vi "Wind_Turbine_1.vi"() -> (5 "Plug in titles":string[](array[string]), 7 "Plug in values":string[](array[string]))   [LabVIEW 2011]
uses:
  Controls/Analysis_info_cluster.ctl
  Controls/Inst_type.ctl
  Controls/Instrument_Array.ctl
  Controls/XY_Plot_Cluster.ctl
  Globals/Meas_global.vi
  Globals/LDA_meas_global_1.vi
  Plug in sub vis/Wind_Turbine_Global.vi
  Globals/Plug_in_data_global.vi
  <vilib>/Analysis/NI_AALBase.lvlib
  <vilib>/Analysis/NI_AALPro.lvlib
panel:
  in  "precision 2":string="3"
  in  "Separation Character 2":string="\t"
  out "L Status Phase lock index 2":i32
  out "Laser Phase lock index 2":i32
  out "XY Graph":cluster{dbl[], dbl[]}[](graph)
  out "WT Revolution Start times":dbl[](array[numeric])
  out "Angle 3":dbl format="%#_3g"
  out "Angle 2":dbl format="%#_3g"
  out "Angle 1":dbl format="%#_3g"
  out "L Status Phase lock index":i32
  out "Laser Status Index":i32
  out "Waveform Graph 3":dbl[](graph)
  out "Laser Phase lock index":i32
  out "Laser Disp Index":i32
  out "Av Variance 3":dbl
  out "Av Variance 2":dbl
  out "Av Variance 1":dbl
  out "slope 3":dbl format="%#_3g"
  out "slope 2":dbl format="%#_3g"
  out "Variance Blade 3":dbl[](graph)
  out "Variance Blade 2":dbl[](graph)
  out "Mean Blade 3":dbl[](graph)
  out "Mean Blade 2":dbl[](graph)
  out "Variance Blade 1":dbl[](graph)
  out "Av Disp 3":dbl
  out "Av Disp 2":dbl
  out "Av Disp 1":dbl
  out "slope 1":dbl format="%#_3g"
  in  "End Cut Deg":dbl
  in  "Start Cut Deg":dbl
  out "Waveform Graph 2":i16[](graph)
  out "Mean Blade 1":dbl[](graph)
  out "Array":i32[](array[numeric])
  in  "Angular Step":dbl=10.0
  in  "Turbine to Phase Lock to":u16(ring) items=["RV (WT1)"]
  in  "Change Dem Voltages?":bool=TRUE
  out "All WTs":dbl[][](array[numeric]) format="%#.2g"
  out "WT trace index":dbl[][](array[numeric])
  in  "precision":string
  in  "Add Phase data to results file":bool
  in  "Separation Character":string="\t"
  in  "Output Directory":path
  in  "Save Phase averaged Profiles":bool
  out "LDA Chs":i32[](array[numeric])
  out "WT Stalled?":bool
  out "Pulse No":i32
  out "Last index":i32
  out "subarray":bool[](array[boolean])
  out "Index":i32[](array[numeric])
  out "Pulses per Rev":i32
  out "Av samples per pulse":i32
  out "Threshold":dbl
  in  "Channel to Phase lock":i32[](listbox)
  out "Last Block No of Revs":i32
  out "Number of Revs":i32
  # "Mean RPM      SD RPM           Max-Min"
  # "Scroll down for Blade angle stats"
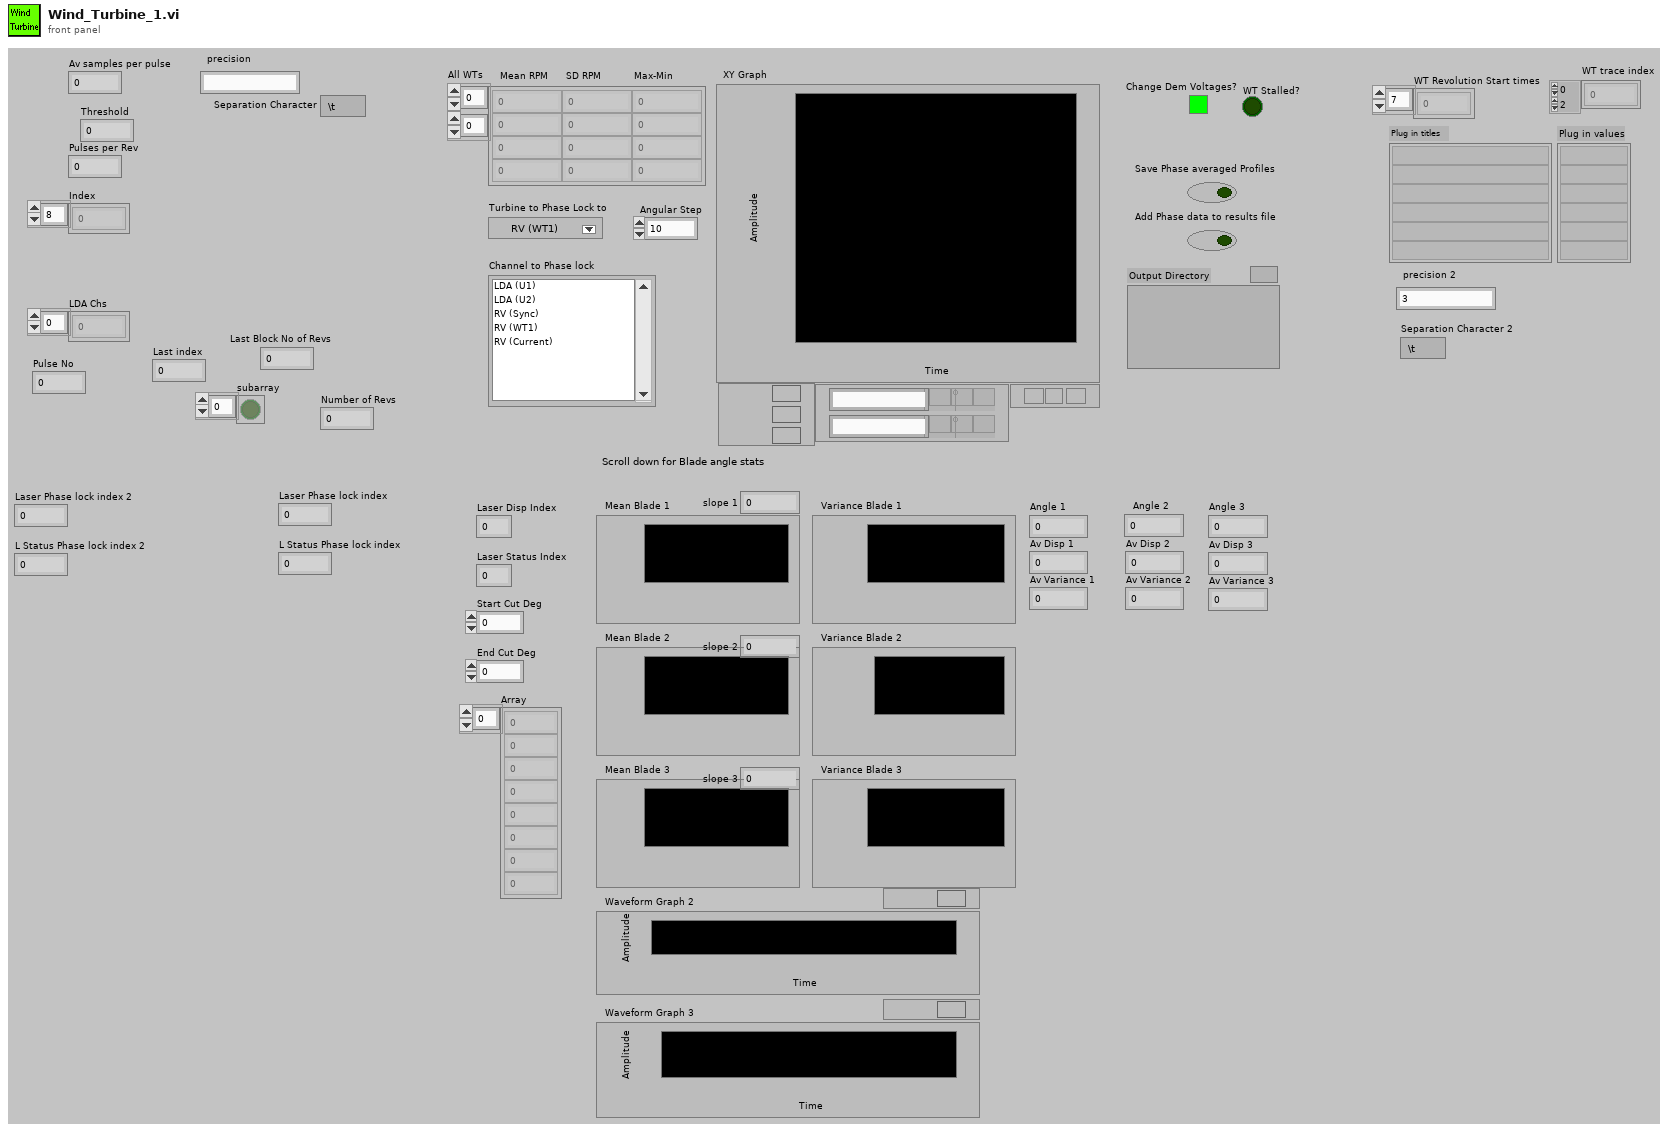
[diagram p1: front panel]
types:
  T1 = typedef "Analysis_info_cluster.ctl" = cluster{"Colour":u32, "Inst type":T2, "Inst name":string, "Symbol":string, "Code name":string, "Extra Info":string, "Inst Array":T3, "Extra Titles":string[], "Extra Values":string[], "Eng Values":dbl[], "Time (ms)":dbl[], "Voltage":dbl[], "U":dbl, "u^2":dbl, "u^3":dbl, "u^4":dbl, "Skew_u":dbl, "Kurt_u":dbl, "Sd Error in Mean":dbl, "% u'/U":dbl, "X":dbl, "Y":dbl, "Z":dbl, "Spectra":T4, "Autocorrelation":T4, "Timescale integral to 25%":dbl, "Sd Error in Variance":dbl, "Calib File":path, "Calib Constants":dbl[], "Histogram":T4, "Output Position":bool, "Full Stats":bool, "Weighting":dbl[], "Av Sampling Rate":dbl, "Av No of Samples":dbl, "Total Meas Time (s)":dbl}
  T2 = typedef "Inst_type.ctl" = enum16{"Propeller anemometer", "Raw voltage", "Pressure Transducer", "Pitot-static tube", "Preston tube", "Hot wire", "Cross wire 1", "Cross wire 2", "Generic Linear", "Generic Polynomial", "Generic BackPoly", "Fast FID", "Thermocouple", "Cold wire", "Pulsed Wire", "LDA Vel", "LDA Tran time", "LDA Arr time"}
  T3 = typedef "Instrument_Array.ctl" = enum16{"PWA", "LDA", "Analogue"}
  T4 = typedef "XY_Plot_Cluster.ctl" = cluster{"First Name":string, "Second Name":string, "X axis name":string, "Y axis name":string, "X array":dbl[], "Y array":dbl[]}
  T5 = typedef "Post_Process.ctl" = enum16{"Take New Data", "Post Process Raw Data File"}
  T6 = cluster{"[0]":bool, "[1]":bool, "[2]":bool, "[3]":bool}
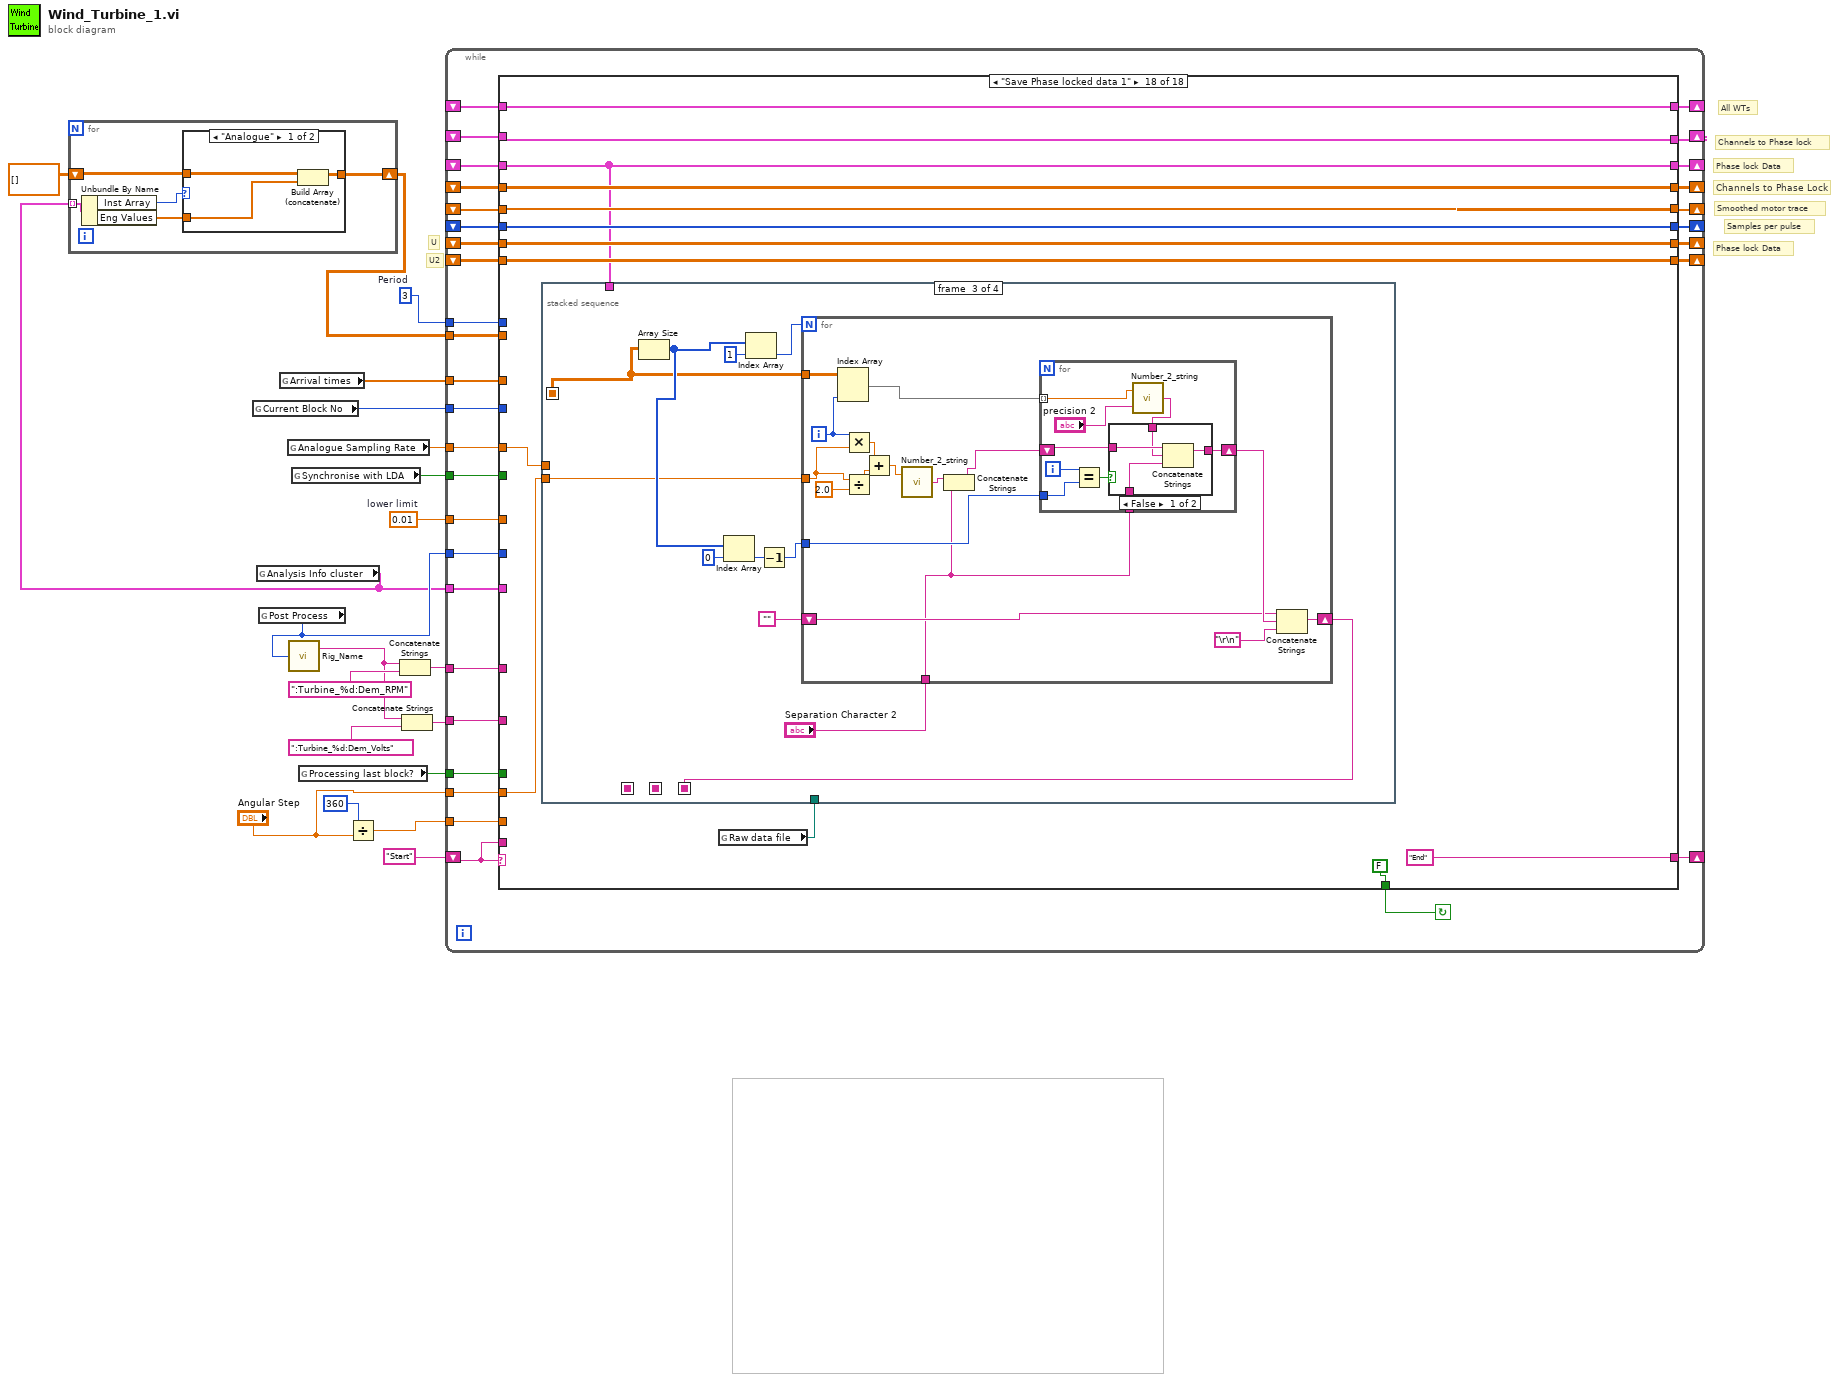
[diagram p0: block diagram]
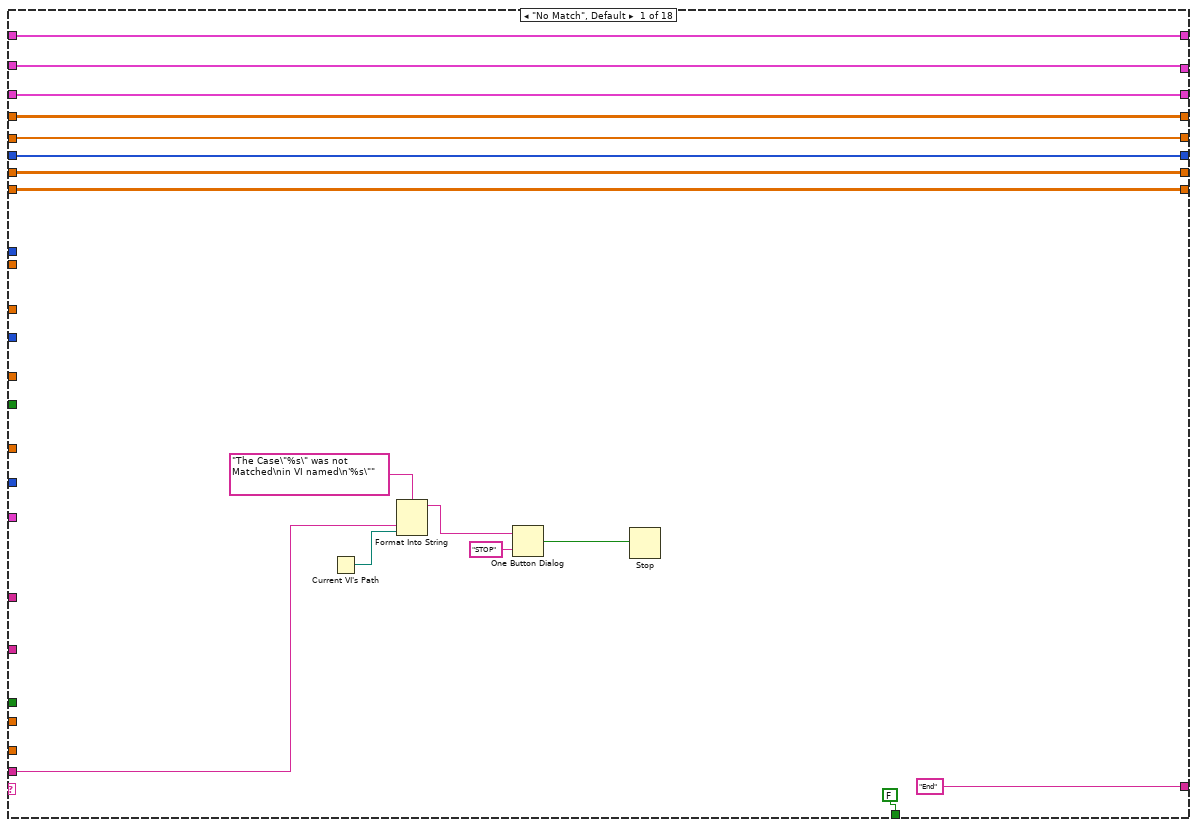
[diagram p3: hidden frame]
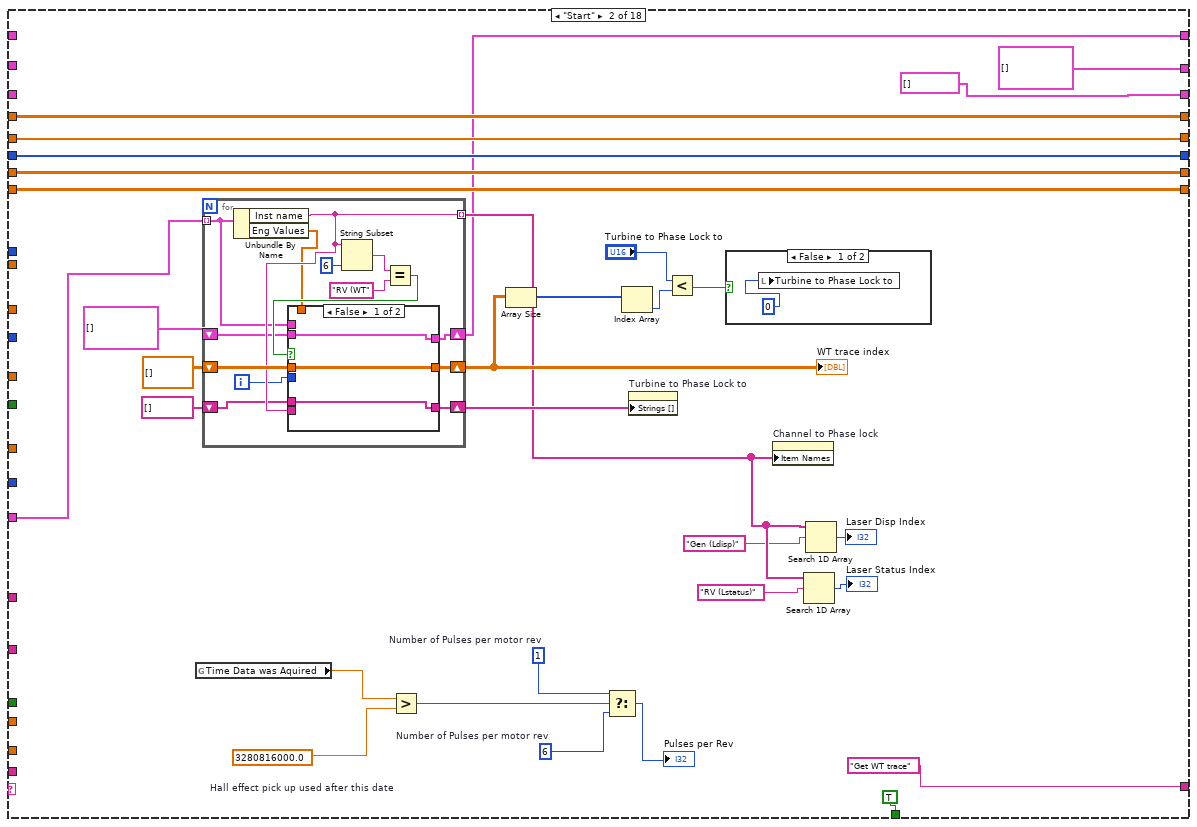
[diagram p4: hidden frame]
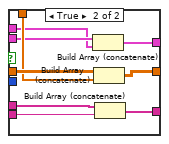
[diagram p6: hidden frame]
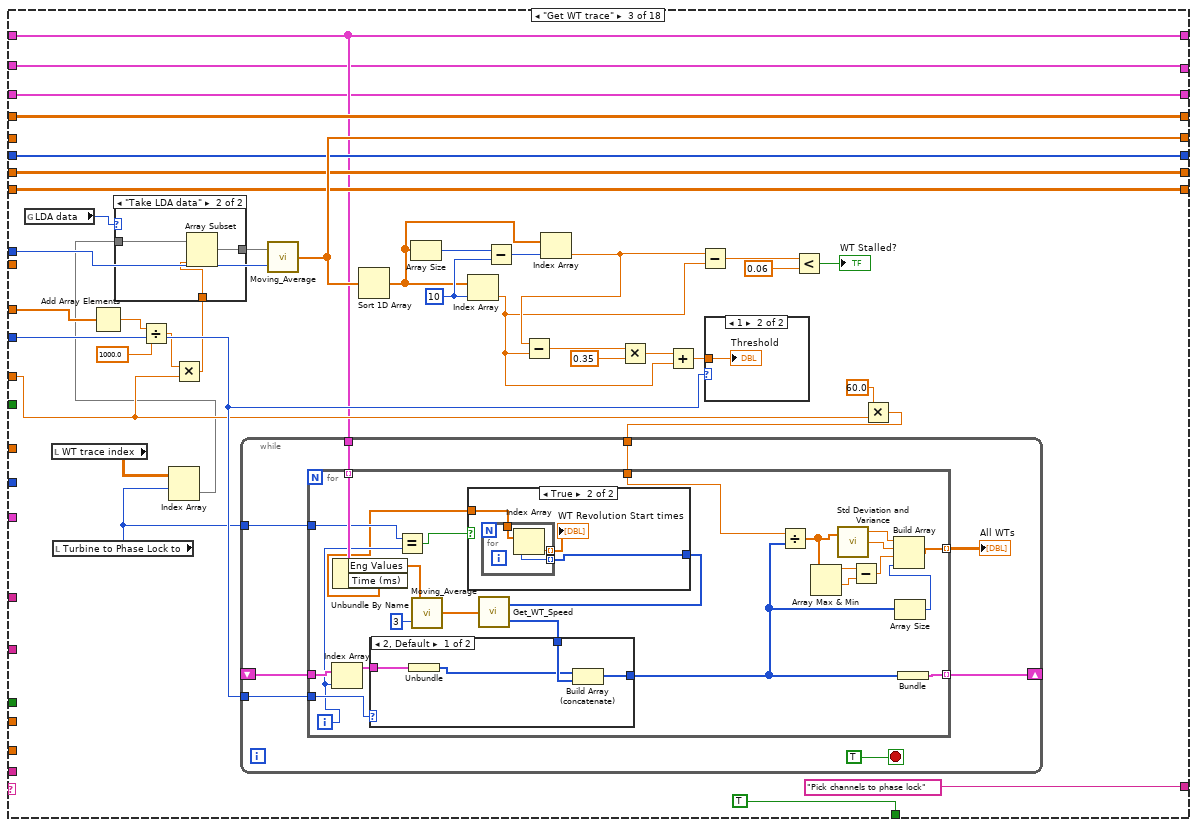
[diagram p7: hidden frame]
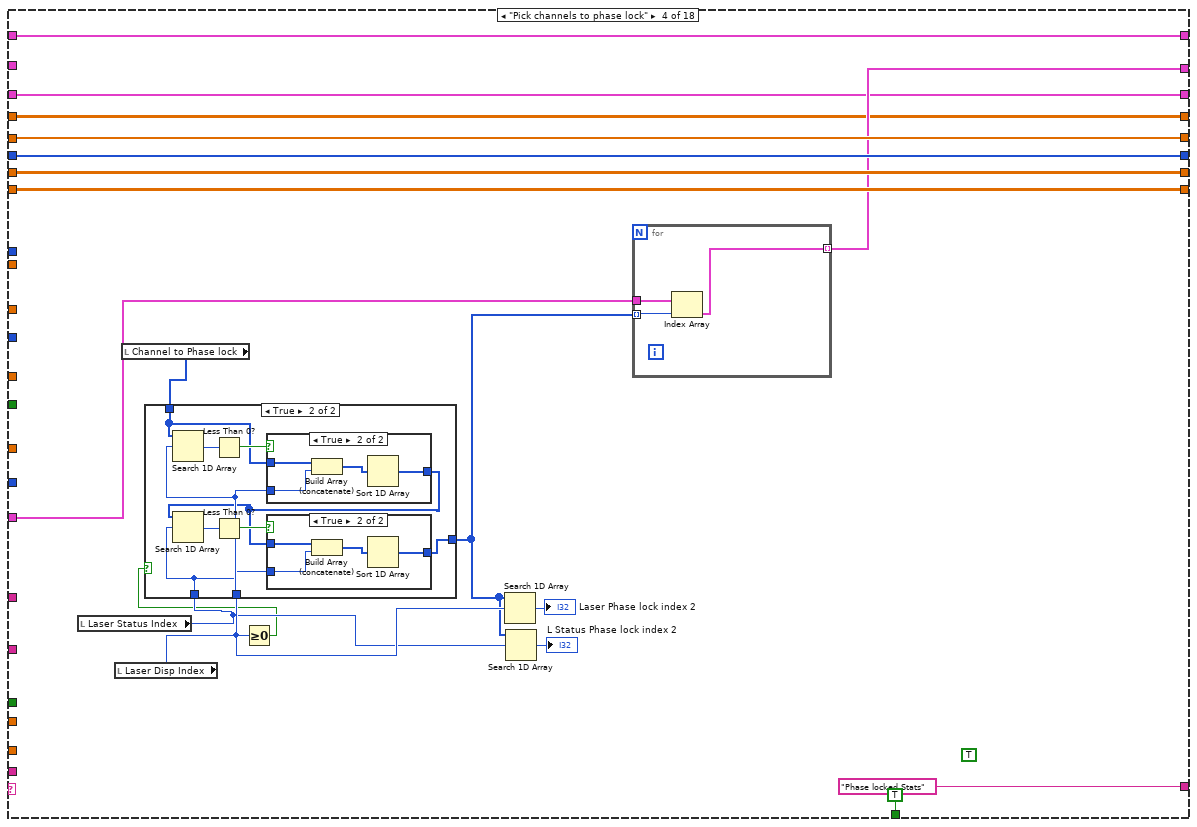
[diagram p12: hidden frame]
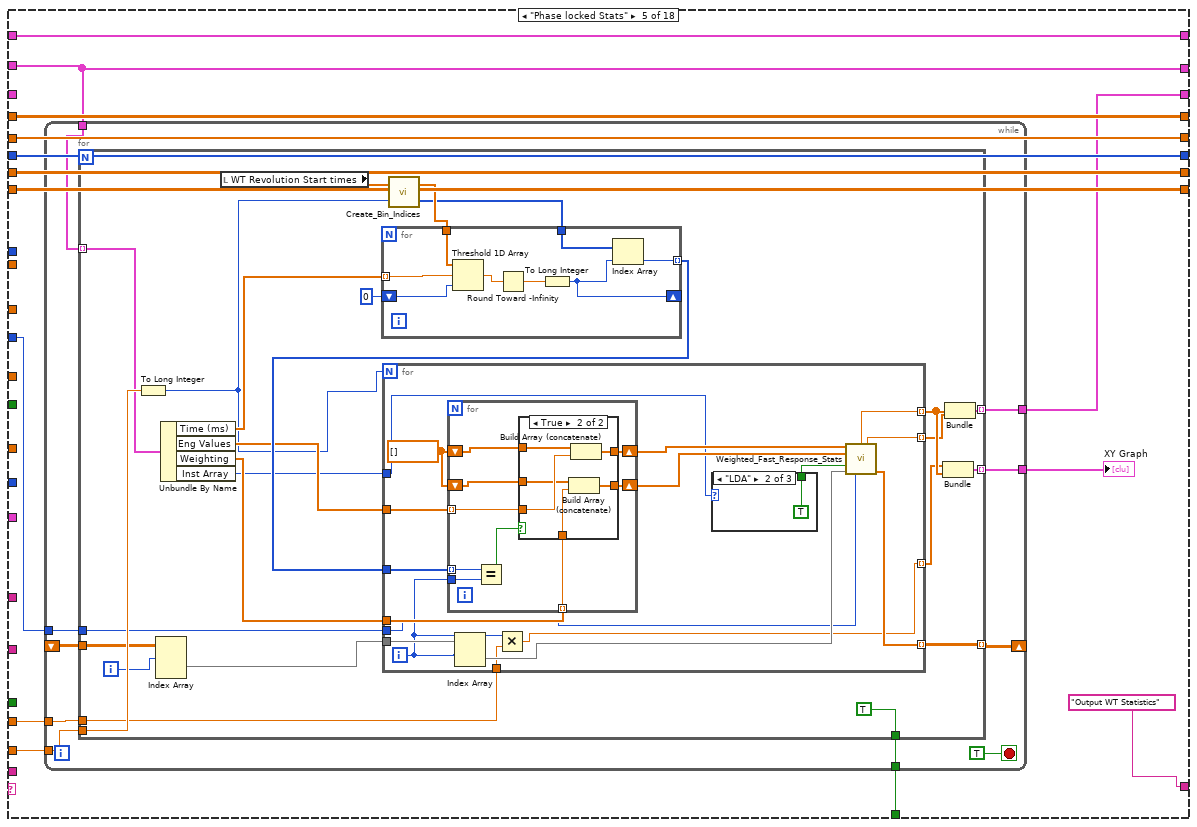
[diagram p16: hidden frame]
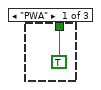
[diagram p17: hidden frame]
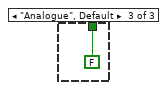
[diagram p18: hidden frame]
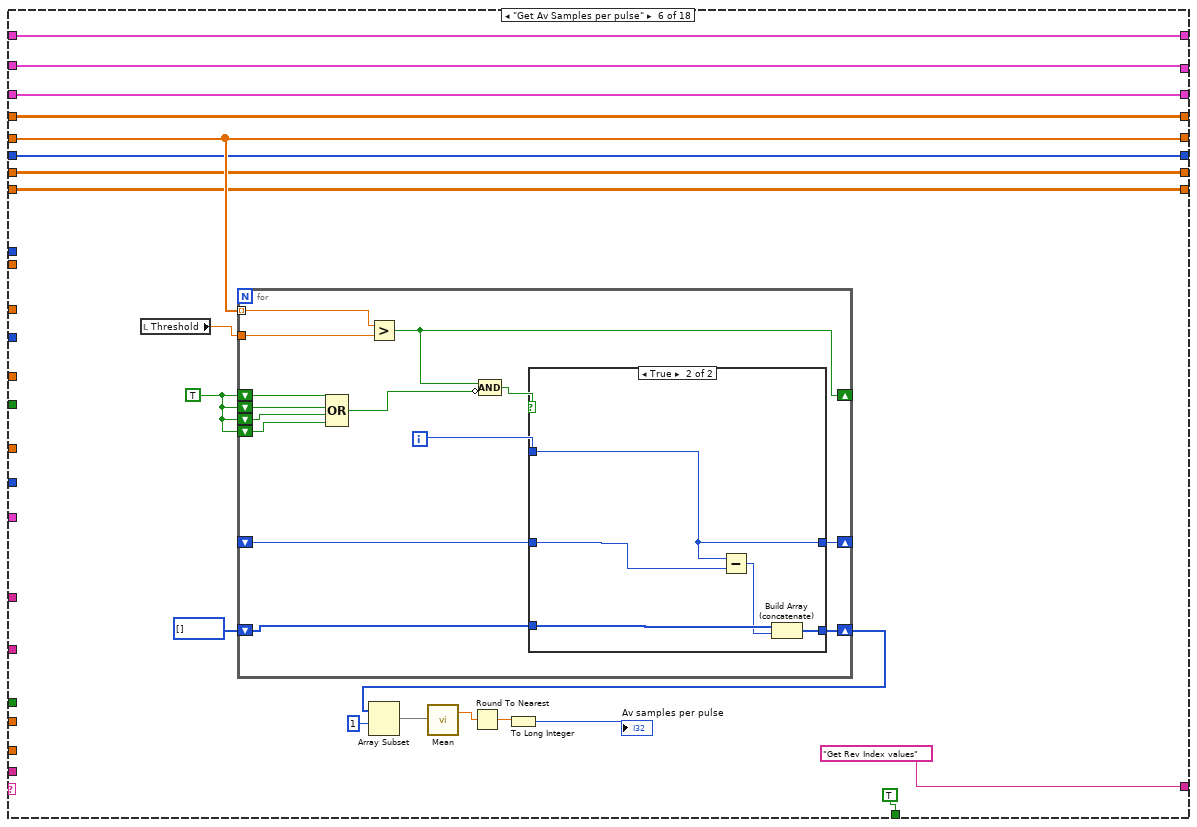
[diagram p20: hidden frame]
diagram:
  w18 = 3  # Period
  w19 = 0.01  # lower limit
  # "Phase lock Data"
  # "Channels to Phase lock"
  # "All WTs"
  # "U"
  # "U2"
  # "Channels to Phase Lock"
  # "Phase lock Data"
  # "Samples per pulse"
  # "Smoothed motor trace"
  n1 = global read "Meas_global.vi" "Current Block No"() -> (w2:i32)
  n2 = global read "Meas_global.vi" "Analysis Info cluster"() -> (w6:T1[])
  n3 = for {
    shift-right: [w22] -> w4
    shift-left: dbl[][] [] -> [w23]
    tunnel: w6 -> [w25] mode=indexing
    n4 = Unbundle By Name(w25) -> ("Inst Array"=w24:T3, "Eng Values"=w21:dbl[])
    n5 = case shown="\"Analogue\"" w24 {
      tunnel: w23 -> [w28 w29]
      tunnel: [w27 w29] -> w22
      tunnel: w21 -> [w26 _]
      frame "Analogue" {
        n6 = Build Array (concatenate)(w28, w26) -> (w27:dbl[][])
      }
      frame "LDA", Default {
      }
    }
  }
  n7 = global read "Meas_global.vi" "Post Process"() -> (w17:T5)
  n8 = global read "LDA_meas_global_1.vi" "Arrival times"() -> (w7:dbl[])
  n9 = global read "Meas_global.vi" "Analogue Sampling Rate"() -> (w20:dbl)
  n10 = call "Rig_Name.vi"("Post Process"=w17) -> ("Rig Setup before dash"=w13:string)  [unwired: 1 out]
  n11 = global read "Meas_global.vi" "Synchronise with LDA"() -> (w11:bool)
  n12 = global read "Meas_global.vi" "Processing last block?"() -> (w9:bool)
  n13 = Divide(x=360, y="Angular Step") -> (x/y=w3:dbl)
  n14 = Concatenate Strings(w13, ":Turbine_%d:Dem_RPM") -> (w12:string)
  n15 = Concatenate Strings(w13, ":Turbine_%d:Dem_Volts") -> (w16:string)
  n16 = while {
    tunnel: w2 -> [w62]
    tunnel: w4 -> [w36]
    shift-right: [w60] -> _
    shift-left: _ -> [w61]
    shift-right: [w59] -> _
    shift-left: _ -> [w58]
    tunnel: w20 -> [w57]
    tunnel: w16 -> [w56]
    tunnel: w12 -> [w55]
    tunnel: w19 -> [w54]
    tunnel: w18 -> [w53]
    tunnel: w17 -> [w52]
    tunnel: w11 -> [w51]
    tunnel: w6 -> [w50]
    shift-right: [w49] -> _
    shift-left: _ -> [w48]
    shift-right: [w47] -> _
    shift-left: "Start" -> [w45]
    tunnel: w9 -> [w44]
    shift-right: [w43] -> _
    shift-left: _ -> [w42]
    tunnel: w3 -> [w41]
    shift-right: [w39] -> _
    shift-left: _ -> [w40]
    tunnel: w7 -> [w38]
    tunnel: "Angular Step" -> [w37]
    shift-right: [w35] -> _
    shift-left: _ -> [w34]
    shift-right: [w32] -> _
    shift-left: _ -> [w33]
    shift-right: [w31] -> _
    shift-left: _ -> [w30]
    stop <- w46 continue-if-true
    n17 = case shown="\"Save Phase locked data 1\"" w45 {
      tunnel: w62 -> [_ _ w152 _ w275 _ w427 _ _ w642 _ _ _ _ _ _ _ _]
      tunnel: w36 -> [_ _ _ _ _ _ _ _ w588 _ _ _ _ _ _ _ _ _]
      tunnel: w61 -> [w70 w98 w162 w237 w270 w362 w405 w528 w595 w638 w701 w749 w934 w979 w1009 w1086 w1103 w1216]
      tunnel: [w70 w98 w162 w237 w270 w362 w405 w528 w595 w637 w701 w749 w934 w979 w1009 w1086 w1103 w1216] -> w60
      tunnel: [w71 w99 w163 w238 w271 w363 w406 w529 w596 w633 w702 w752 w932 w977 w1017 w1087 w1108 w1221] -> w59
      tunnel: w58 -> [w71 w99 w163 w238 w271 w363 w406 w529 w596 w624 w702 w752 w932 w977 w1017 w1087 w1108 w1221]
      tunnel: w57 -> [_ _ w147 _ _ _ _ _ w591 _ _ w753 _ _ _ _ w1107 w1220]
      tunnel: w56 -> [_ _ _ _ _ _ _ _ _ _ _ _ w939 w975 _ _ _ _]
      tunnel: w55 -> [_ _ _ _ _ _ _ _ _ _ _ _ w938 w950 _ _ _ _]
      tunnel: w54 -> [_ _ _ _ _ _ _ _ _ _ _ _ _ _ _ _ _ _]
      tunnel: w53 -> [_ _ w174 _ _ _ _ _ _ _ _ _ _ _ _ _ _ _]
      tunnel: w52 -> [_ _ _ _ _ _ _ _ _ _ _ _ w937 _ _ _ _ _]
      tunnel: w51 -> [_ _ _ _ _ _ w412 _ _ _ _ _ _ _ _ _ _ _]
      tunnel: w50 -> [_ w103 _ w229 _ _ _ w532 _ _ _ _ _ _ _ _ _ _]
      tunnel: [w72 w100 w167 w239 w272 w364 w407 w530 w597 w632 w703 w751 w935 w980 w1018 w1088 w1109 w1222] -> w49
      tunnel: w48 -> [w72 w100 _ w239 w272 w364 w407 w530 w597 w632 w703 w751 w935 w980 w1018 w1088 w1109 w1222]
      tunnel: ["End" "Get WT trace" "Pick channels to phase lock" "Phase locked Stats" ("f") "Output WT Statistics" "Get Rev Index values" "Prepare Phase Lock Channels" w524 "WT trace Phase locked data" ("f") "Output WT Statistics" w707 w743 w936 "End" ("f") "Check Folder Name" "Save Phase locked data 1" "End" "End"] -> w47
      tunnel: [FALSE ("Change Control Voltage?") TRUE ("Processing last block?") TRUE TRUE ("Change Control Voltage?") w267 TRUE ("Processing last block?") TRUE ("Change Control Voltage?") TRUE ("Change Control Voltage?") TRUE ("Change Control Voltage?") TRUE ("Change Control Voltage?") TRUE ("Change Control Voltage?") w744 w930 FALSE ("Change Control Voltage?") w1014 w1078 FALSE ("Change Control Voltage?") FALSE ("Change Control Voltage?")] -> w46
      tunnel: w45 -> [w73 _ _ _ _ _ _ _ _ _ _ _ _ _ _ _ _ _]
      tunnel: w44 -> [_ _ _ _ _ _ _ _ _ _ _ w745 w929 _ w1012 _ _ _]
      tunnel: [w67 w97 w161 w226 w273 w361 w402 w511 w577 w628 w704 w750 w933 w978 w1016 w1085 w1106 w1219] -> w43
      tunnel: w42 -> [w67 w97 w161 w226 w273 w361 w402 _ w579 w628 w704 w750 w933 w978 w1016 w1085 w1106 w1219]
      tunnel: w41 -> [_ _ _ _ w277 _ _ _ _ w627 _ w748 _ _ w1010 _ w1101 _]
      tunnel: w40 -> [w66 w96 w160 w236 w269 w360 w401 w520 w578 w621 w700 w746 w931 w976 w1008 w1076 w1102 w1215]
      tunnel: [w66 w96 w160 w236 w269 w360 w401 w520 w578 w620 w700 w746 w931 w976 w1008 w1076 w1102 w1215] -> w39
      tunnel: w38 -> [_ _ w150 _ _ _ _ _ w576 _ _ _ _ _ _ _ _ _]
      tunnel: w37 -> [_ _ _ _ w276 _ _ _ _ _ _ w747 _ _ _ _ _ w1211]
      tunnel: [w65 w81 w139 w240 w274 w359 w399 w510 w575 w616 w699 w742 w928 w949 w1007 w1075 w1100 w1214] -> w35
      tunnel: w34 -> [w65 _ w139 w240 w274 w359 w399 w510 w575 w616 w699 w742 w928 w949 w1007 w1075 w1100 w1214]
      tunnel: w33 -> [w64 _ w138 _ w268 w358 w398 w509 w574 w615 w698 w741 w927 w948 w1006 w1074 w1099 w1213]
      tunnel: [w64 T1[] [] w138 w227 w268 w358 w398 w509 w574 w615 w698 w741 w927 w948 w1006 w1074 w1099 w1213] -> w32
      tunnel: [w63 cluster{dbl[], dbl[]}[] [] w137 w223 w265 w357 w397 w508 w573 w614 w697 w740 w926 w947 w1005 w1073 w1098 w1212] -> w31
      tunnel: w30 -> [w63 _ w137 w223 _ w357 w397 w508 w573 w614 w697 w740 w926 w947 w1005 w1073 w1098 w1212]
      frame "No Match", Default {
        n18 = Current VI's Path() -> (path=w74:path)
        n19 = Format Into String(format string="The Case\"%s\" was not Matched\nin VI named\n'%s\"" ("Format String"), w73, w74) -> (resulting string=w77:string)  [unwired: 2 in, 1 out]
        n20 = One Button Dialog(message=w77, button name ("OK")="STOP") -> (true=w75:bool)
        n21 = Stop(stop? (T)=w75) -> ()
      }
      frame "Start" {
        w104 = 6  # Number of Pulses per motor rev
        w105 = 1  # Number of Pulses per motor rev
        w107 = 3280816000.0  # Hall effect pick up used after this date
        n22 = global read "Meas_global.vi" "Time Data was Aquired"() -> (w108:dbl)
        n23 = for {
          tunnel: w103 -> [w112] mode=indexing
          tunnel: [w118] -> w88 mode=indexing
          shift-right: [w119] -> w93
          shift-left: dbl[][] [] -> [w120]
          shift-right: [w117] -> w94
          shift-left: string[] [] -> [w116]
          shift-right: [w111] -> w81
          shift-left: T1[] [] -> [w113]
          i -> [w115]
          n24 = Unbundle By Name(w112) -> ("Inst name"=w118:string, "Eng Values"=w114:dbl[])
          n25 = String Subset(string=w118, length (rest)=6 ("length (rest)")) -> (substring=w122:string)  [unwired: 1 out]
          n26 = Equal?(x=w122, y="RV (WT") -> (x = y?=w121:bool)
          n27 = case shown="False" w121 {
            tunnel: w120 -> [w127 w136]
            tunnel: [w127 w131] -> w119
            tunnel: w115 -> [_ _]
            tunnel: w118 -> [_ w135]
            tunnel: [w126 w134] -> w117
            tunnel: w116 -> [w126 w133]
            tunnel: w114 -> [_ w132]
            tunnel: w113 -> [w125 w130]
            tunnel: w112 -> [_ w129]
            tunnel: [w125 w128] -> w111
            frame False {
            }
            frame True {
              n28 = Build Array (concatenate)(w130, w129) -> (w128:T1[])
              n29 = Build Array (concatenate)(w136, w132) -> (w131:dbl[][])
              n30 = Build Array (concatenate)(w133, w135) -> (w134:string[])
            }
          }
        }
        "WT trace index" <- w93
        n31 = Greater?(x=w108, y=w107) -> (0:w106:bool)
        n32 = Array Size(array=w93) -> (size(s)=w84:i32[])
        n33 = Select(t=w105, s=w106, f=w104) -> (s? t:f=→"Pulses per Rev":i32)
        n34 = Index Array(array=w84) -> (element=w83:i32)  [unwired: 1 in]
        n35 = property on="Turbine to Phase Lock to" class="Ring (strict)"("Strings []"=w94) -> ()  [unwired: 2 in, 2 out]
        n36 = Less?(x="Turbine to Phase Lock to", y=w83) -> (x < y?=w91:bool)
        n37 = case shown="False" w91 {
          frame False {
            n38 = local write "Turbine to Phase Lock to"(0) -> ()
          }
          frame True {
          }
        }
        n39 = property on="Channel to Phase lock" class="LstBox (strict)"("Item Names"=w88) -> ()  [unwired: 2 in, 2 out]
        n40 = Search 1D Array(1D array=w88, element="RV (Lstatus)") -> (index of element=→"Laser Status Index":i32)  [unwired: 1 in]
        n41 = Search 1D Array(1D array=w88, element="Gen (Ldisp)") -> (index of element=→"Laser Disp Index":i32)  [unwired: 1 in]
      }
      frame "Get WT trace" {
        w172 = 10 ("index")
        n42 = global read "Meas_global.vi" "LDA data"() -> (w143:enum16{"No LDA data", "Take LDA data"})
        n43 = local read "WT trace index"() -> (w142:dbl[][])
        n44 = local read "Turbine to Phase Lock to"() -> (w140:u16)
        n45 = Add Array Elements(numeric array=w150) -> (sum=w149:dbl)
        n46 = Divide(x=w149, y=1000.0) -> (x/y=w146:dbl)
        n47 = Index Array(array=w142, index (row)=w140) -> (element=w141:dbl[])  [unwired: 1 in]
        n48 = Multiply(x=w146, y=w147) -> (x*y=w144:dbl)
        n49 = case shown="\"Take LDA data\"" w143 {
          tunnel: w141 -> [w175 w178]
          tunnel: [w175 w177] -> w145
          tunnel: w144 -> [_ w176]
          frame "No LDA data" {
          }
          frame "Take LDA data" {
            n50 = Array Subset(array=w178, length=w176) -> (w177:dbl[])  [unwired: 1 in]
          }
        }
        n51 = call "Moving_Average.vi"("Period"=w174, "Input Array"=w145) -> ("N+1-Period"=w167:dbl[])
        n52 = Sort 1D Array(array=w167) -> (sorted array=w170:dbl[])
        n53 = Array Size(array=w170) -> (size(s)=w173:i32)
        n54 = Index Array(array=w170, index=w172) -> (element=w153:dbl)
        n55 = Subtract(x=w173, y=w172) -> (x-y=w171:i32)
        n56 = Index Array(array=w170, index=w171) -> (element=w154:dbl)
        n57 = Subtract(x=w154, y=w153) -> (x-y=w157:dbl)
        n58 = Multiply(x=w157, y=0.35) -> (x*y=w155:dbl)
        n59 = Add(x=w155, y=w153) -> (x+y=w151:dbl)
        n60 = Subtract(x=w154, y=w153) -> (x-y=w168:dbl)
        n61 = case shown="1" w152 {
          tunnel: w151 -> [_ w179]
          frame 0, Default {
          }
          frame 1 {
            "Threshold" <- w179
          }
        }
        n62 = Less?(x=w168, y=0.06) -> (x < y?=→"WT Stalled?":bool)
        n63 = Multiply(x=60.0, y=w147) -> (x*y=w158:dbl)
        n64 = while {
          tunnel: w152 -> [w187]
          shift-right: [w182] -> _
          shift-left: _ -> [w186]
          tunnel: w158 -> [w185]
          tunnel: w139 -> [w181]
          tunnel: w140 -> [w180]
          stop <- TRUE stop-if-true
          n65 = for {
            tunnel: w187 -> [w210]
            tunnel: w186 -> [w200]
            tunnel: w185 -> [w208]
            tunnel: [w201] -> w183 mode=indexing
            tunnel: [w196] -> w182 mode=indexing
            tunnel: w181 -> [w195] mode=indexing
            tunnel: w180 -> [w190]
            i -> [w191]
            n66 = Index Array(array=w200, index=w191) -> (element=w199:cluster{"Samples per pulse":i32[]})
            n67 = Unbundle By Name(w195) -> ("Eng Values"=w194:dbl[], "Time (ms)"=w188:dbl[])
            n68 = Equal?(x=w190, y=w191) -> (x = y?=w189:bool)
            n69 = call "Moving_Average.vi"("Period"=3, "Input Array"=w194) -> ("N+1-Period"=w211:dbl[])
            n70 = call "Get_WT_Speed.vi"("Opto Trace"=w211) -> ("Start Cycle Index"=w192:i32[], "Samples per pulse"=w209:i32[])
            n71 = case shown="2, Default" w210 {
              tunnel: [w220 w222] -> w197
              tunnel: w209 -> [w221 w222]
              tunnel: w199 -> [w219 _]
              frame 2, Default {
                n72 = Unbundle(w219) -> ("Samples per pulse"=w218:i32[])
                n73 = Build Array (concatenate)(w218, w221) -> (w220:i32[])
              }
              frame 1 {
              }
            }
            n74 = case shown="True" w189 {
              tunnel: w192 -> [_ w214]
              tunnel: w188 -> [_ w213]
              frame False {
              }
              frame True {
                n75 = for {
                  tunnel: w214 -> [w217] mode=indexing
                  tunnel: w213 -> [w216]
                  tunnel: [w215] -> w212 mode=indexing
                  n76 = Index Array(array=w216, index=w217) -> (element=w215:dbl)
                }
                "WT Revolution Start times" <- w212
              }
            }
            n77 = Divide(x=w208, y=w197) -> (x/y=w205:dbl[])
            n78 = Array Max & Min(array=w205) -> (max value=w207:dbl, min value=w206:dbl)  [unwired: 2 out]
            n79 = call <vilib>:"Std Deviation and Variance.vi"("X"=w205) -> ("mean"=w204:dbl, "standard deviation"=w203:dbl)  [unwired: 1 in, 1 out]
            n80 = Subtract(x=w207, y=w206) -> (x-y=w202:dbl)
            n81 = Array Size(array=w197) -> (size(s)=w198:i32)
            n82 = Build Array(w204, w203, w202, w198) -> (w201:dbl[])
            n83 = Bundle("Samples per pulse"=w197) -> (w196:cluster{"Samples per pulse":i32[]})  [unwired: 1 in]
          }
          "All WTs" <- w183
        }
      }
      frame "Pick channels to phase lock" {
        (unwired) TRUE ("Change Control Voltage?")
        n84 = local read "Laser Status Index"() -> (w230:i32)
        n85 = local read "Laser Disp Index"() -> (w233:i32)
        n86 = local read "Channel to Phase lock"() -> (w225:i32[])
        n87 = Greater Or Equal To 0?(x=w233) -> (x >= 0?=w228:bool)
        n88 = case shown="True" w228 {
          tunnel: w225 -> [w241 w248]
          tunnel: w233 -> [_ w247]
          tunnel: [w241 w244] -> w224
          tunnel: w230 -> [_ w242]
          frame False {
          }
          frame True {
            n89 = Search 1D Array(1D array=w248, element=w247) -> (index of element=w250:i32)  [unwired: 1 in]
            n90 = Less Than 0?(x=w250) -> (x < 0?=w249:bool)
            n91 = case shown="True" w249 {
              tunnel: w248 -> [w256 w260]
              tunnel: w247 -> [_ w259]
              tunnel: [w256 w257] -> w243
              frame False {
              }
              frame True {
                n92 = Build Array (concatenate)(w260, w259) -> (w258:i32[])
                n93 = Sort 1D Array(array=w258) -> (sorted array=w257:i32[])
              }
            }
            n94 = Search 1D Array(1D array=w243, element=w242) -> (index of element=w245:i32)  [unwired: 1 in]
            n95 = Less Than 0?(x=w245) -> (x < 0?=w246:bool)
            n96 = case shown="True" w246 {
              tunnel: w243 -> [w251 w255]
              tunnel: w242 -> [_ w254]
              tunnel: [w251 w252] -> w244
              frame False {
              }
              frame True {
                n97 = Build Array (concatenate)(w255, w254) -> (w253:i32[])
                n98 = Sort 1D Array(array=w253) -> (sorted array=w252:i32[])
              }
            }
          }
        }
        n99 = Search 1D Array(1D array=w224, element=w233) -> (index of element=→"Laser Phase lock index 2":i32)  [unwired: 1 in]
        n100 = Search 1D Array(1D array=w224, element=w230) -> (index of element=→"L Status Phase lock index 2":i32)  [unwired: 1 in]
        n101 = for {
          tunnel: w224 -> [w263] mode=indexing
          tunnel: w229 -> [w262]
          tunnel: [w261] -> w227 mode=indexing
          n102 = Index Array(array=w262, index=w263) -> (element=w261:T1)
        }
      }
      frame "Phase locked Stats" {
        n103 = while {
          tunnel: w277 -> [w287]
          tunnel: w276 -> [w286]
          tunnel: w275 -> [w285]
          tunnel: w268 -> [w279]
          tunnel: [w284] -> w267
          tunnel: [w283] -> w264
          shift-right: [w282] -> _
          shift-left: _ -> [w280]
          tunnel: [w278] -> w265
          stop <- TRUE stop-if-true
          n104 = for {
            tunnel: w287 -> [w306]
            tunnel: w286 -> [w305]
            tunnel: w285 -> [w304]
            tunnel: w279 -> [w300] mode=indexing
            tunnel: [TRUE] -> w284
            tunnel: [w297] -> w283 mode=indexing
            tunnel: [w296] -> w282 mode=indexing
            tunnel: w280 -> [w295]
            tunnel: [w289] -> w278 mode=indexing
            i -> [w294]
            n105 = To Long Integer(number=w306) -> (32bit integer=w288:i32)
            n106 = Index Array(array=w295, index (dim 0)=w294) -> (element=w293:dbl[][])  [unwired: 2 in]
            n107 = Unbundle By Name(w300) -> ("Time (ms)"=w299:dbl[], "Eng Values"=w303:dbl[], "Weighting"=w302:dbl[], "Inst Array"=w301:T3)
            n108 = local read "WT Revolution Start times"() -> (w310:dbl[])
            n109 = call "Create_Bin_Indices.vi"("No Of Bins"=w288, "Cycle Start TIme"=w310) -> ("Bin Number"=w308:i32[], "Bin Start Time"=w309:dbl[])
            n110 = for {
              tunnel: w309 -> [w356]
              tunnel: w299 -> [w355] mode=indexing
              shift-right: [w352] -> _
              shift-left: 0 -> [w349]
              tunnel: w308 -> [w353]
              tunnel: [w351] -> w307 mode=indexing
              n111 = Threshold 1D Array(1:w349, 2:w355, 3:w356) -> (0:w354:dbl)
              n112 = Round Toward -Infinity(1:w354) -> (0:w350:dbl)
              n113 = To Long Integer(number=w350) -> (32bit integer=w352:i32)
              n114 = Index Array(array=w353, index=w352) -> (element=w351:i32)
            }
            n115 = for {
              N: w288 -> [_]
              tunnel: w307 -> [w328]
              tunnel: w303 -> [w327]
              tunnel: w302 -> [w325]
              tunnel: w293 -> [w322]
              tunnel: [w320] -> w296 mode=indexing
              tunnel: w304 -> [w319]
              tunnel: [w317] -> w292 mode=indexing
              tunnel: w305 -> [w315]
              tunnel: [w314] -> w291 mode=indexing
              tunnel: w301 -> [w313]
              tunnel: [w312] -> w290 mode=indexing
              i -> [w316]
              w326 = dbl[] []
              n116 = for {
                tunnel: w316 -> [w340]
                tunnel: w328 -> [w339] mode=indexing
                shift-right: [w335] -> w323
                shift-left: w326 -> [w337]
                tunnel: w327 -> [w336] mode=indexing
                shift-right: [w334] -> w324
                shift-left: w326 -> [w333]
                tunnel: w325 -> [w332] mode=indexing
                n117 = Equal?(x=w339, y=w340) -> (x = y?=w338:bool)
                n118 = case shown="True" w338 {
                  tunnel: w337 -> [w342 w348]
                  tunnel: w336 -> [_ w347]
                  tunnel: [w342 w346] -> w335
                  tunnel: w333 -> [w341 w344]
                  tunnel: [w341 w345] -> w334
                  tunnel: w332 -> [_ w343]
                  frame False {
                  }
                  frame True {
                    n119 = Build Array (concatenate)(w344, w343) -> (w345:dbl[])
                    n120 = Build Array (concatenate)(w348, w347) -> (w346:dbl[])
                  }
                }
              }
              n121 = Index Array(array=w322, index (row)=w316) -> (element=w321:dbl[])  [unwired: 1 in]
              n122 = Multiply(x=w316, y=w315) -> (x*y=w314:dbl)
              n123 = case shown="\"LDA\"" w313 {
                tunnel: [TRUE ("Use Weighting?") TRUE ("Use Weighting?") FALSE ("Use Weighting?")] -> w318
                frame "PWA" {
                }
                frame "LDA" {
                }
                frame "Analogue", Default {
                }
              }
              n124 = call "Weighted_Fast_Response_Stats.vi"("U"=w323, "Weighting"=w324, "Use Weighting?"=w318, "Shift in"=w321, "Block No"=w319) -> ("U"=w317:dbl, "u^2"=w312:dbl, "Shift out"=w320:dbl[])  [unwired: 3 in, 5 out]
            }
            n125 = Bundle(w291, w292) -> (w297:cluster{dbl[], dbl[]})  [unwired: 1 in]
            n126 = Bundle(w292, w290) -> (w289:cluster{dbl[], dbl[]})  [unwired: 1 in]
          }
        }
        "XY Graph" <- w264
      }
      frame "Get Av Samples per pulse" {
        w373 = TRUE
        n127 = local read "Threshold"() -> (w367:dbl)
        n128 = for {
          shift-right: [w376] -> _
          shift-left: w373 -> [w381]
          shift-right: [w386] -> _
          shift-left: _ -> [w385]
          tunnel: w364 -> [w389] mode=indexing
          tunnel: w367 -> [w388]
          shift-right: [w383] -> w372
          shift-left: i32[] [] -> [w384]
          shift-left: w373 -> [w380]
          shift-left: w373 -> [w379]
          shift-left: w373 -> [w377]
          i -> [w382]
          n129 = Compound Arithmetic op=OR(w381, w380, w379, w377) -> (w378:bool)
          n130 = Greater?(x=w389, y=w388) -> (0:w376:bool)
          n131 = Compound Arithmetic op=AND(w376, invert w378) -> (w387:bool)
          n132 = case shown="True" w387 {
            tunnel: [w391 w394] -> w386
            tunnel: w382 -> [_ w394]
            tunnel: w385 -> [w391 w393]
            tunnel: w384 -> [w390 w396]
            tunnel: [w390 w395] -> w383
            frame False {
            }
            frame True {
              n133 = Subtract(x=w394, y=w393) -> (x-y=w392:i32)
              n134 = Build Array (concatenate)(w396, w392) -> (w395:i32[])
            }
          }
        }
        n135 = Array Subset(array=w372, index=1) -> (w370:i32[])  [unwired: 1 in]
        n136 = call <vilib>:"Mean.vi"("X"=w370) -> ("mean"=w369:dbl)  [unwired: 1 out]
        n137 = Round To Nearest(number=w369) -> (nearest integer value=w368:dbl)
        n138 = To Long Integer(number=w368) -> (32bit integer=→"Av samples per pulse":i32)
      }
      frame "Get Rev Index values" {
        n139 = case shown="2, Default" w427 {
          tunnel: [w429 -1] -> w426
          tunnel: [w430 0] -> w424
          tunnel: [w436 w445] -> w419
          tunnel: [w435 w445] -> w418
          tunnel: [w434 w445] -> w417
          tunnel: [w433 w445] -> w416
          tunnel: [FALSE TRUE] -> w415
          tunnel: w412 -> [w431 _]
          frame 2, Default {
            n140 = case shown="False" w431 {
              tunnel: [w441 w444] -> w436
              tunnel: [w440 w444] -> w435
              tunnel: [w439 w444] -> w434
              tunnel: [w438 w444] -> w433
              frame False {
                n141 = local read "subarray"() -> (w437:bool[])
                n142 = Reverse 1D Array(array=w437) -> (reversed array=w443:bool[])
                n143 = Array To Cluster(array=w443) -> (cluster=w442:T6)
                n144 = Unbundle(w442) -> ("[0]"=w441:bool, "[1]"=w440:bool, "[2]"=w439:bool, "[3]"=w438:bool)
              }
              frame True {
                w444 = TRUE ("[0]")
              }
            }
            n145 = local read "Last index"() -> (w430:i32)
            n146 = local read "Pulse No"() -> (w429:i32)
          }
          frame 1 {
            w445 = TRUE
          }
        }
        n147 = local read "Pulses per Rev"() -> (w409:i32)
        n148 = local read "Av samples per pulse"() -> (w410:i32)
        n149 = local read "Threshold"() -> (w411:dbl)
        n150 = for {
          shift-right: [w456] -> _
          shift-left: w419 -> [w460]
          shift-right: [w467] -> w413
          shift-left: w424 -> [w464]
          tunnel: w407 -> [w470] mode=indexing
          tunnel: w411 -> [w469]
          shift-right: [w465] -> w408
          shift-left: w426 -> [w466]
          shift-right: [w462] -> w400
          shift-left: i32[] [] -> [w463]
          tunnel: [w461] -> w414
          shift-left: w418 -> [w459]
          shift-left: w417 -> [w458]
          tunnel: [w456] -> w421 mode=indexing
          shift-left: w416 -> [w455]
          tunnel: w410 -> [w454]
          tunnel: w415 -> [w450]
          tunnel: w409 -> [w453]
          i -> [w461]
          n151 = Greater?(x=w470, y=w469) -> (0:w456:bool)
          n152 = Equal?(x=1, y=w453) -> (x = y?=w451:bool)
          n153 = Compound Arithmetic op=OR(w460, w459, w458, w455) -> (w457:bool)
          n154 = Or(x=w450, y=w451) -> (x .or. y?=w449:bool)
          n155 = Compound Arithmetic op=AND(w456, invert w457) -> (w468:bool)
          n156 = case shown="True" w468 {
            tunnel: [w473 w483] -> w467
            tunnel: w461 -> [_ w489]
            tunnel: w466 -> [w472 w492]
            tunnel: [w472 w491] -> w465
            tunnel: w464 -> [w473 w482]
            tunnel: w463 -> [w471 w481]
            tunnel: [w471 w490] -> w462
            tunnel: w454 -> [_ w487]
            tunnel: w449 -> [_ w476]
            tunnel: w453 -> [_ w475]
            frame False {
            }
            frame True {
              n157 = Subtract(x=w489, y=w482) -> (x-y=w488:i32)
              n158 = Subtract(x=w488, y=w487) -> (x-y=w486:i32)
              n159 = Array Size(array=w481) -> (size(s)=w479:i32)
              n160 = Absolute Value(x=w486) -> (abs(x)=w485:i32)
              n161 = Equal To 0?(x=w479) -> (x = 0?=w478:bool)
              n162 = And(x=w476, y=w478) -> (x .and. y?=w477:bool)
              n163 = Less?(x=w485, y=35) -> (x < y?=w474:bool)
              n164 = Or(x=w474, y=w477) -> (x .or. y?=w480:bool)
              n165 = case shown="True" w480 {
                tunnel: w492 -> [w495 w503]
                tunnel: [w495 w502] -> w491
                tunnel: w481 -> [w494 w499]
                tunnel: [w494 w498] -> w490
                tunnel: w489 -> [_ w497]
                tunnel: [w493 w497] -> w483
                tunnel: w482 -> [w493 _]
                tunnel: w475 -> [_ w496]
                frame False {
                }
                frame True {
                  n166 = Increment(x=w503) -> (x+1=w502:i32)
                  n167 = Quotient & Remainder(x=w502, y=w496) -> (x-y*floor(x/y)=w501:i32)  [unwired: 1 out]
                  n168 = Equal To 0?(x=w501) -> (x = 0?=w500:bool)
                  n169 = case shown="True" w500 {
                    tunnel: w499 -> [w504 w507]
                    tunnel: w497 -> [_ w506]
                    tunnel: [w504 w505] -> w498
                    frame False {
                    }
                    frame True {
                      n170 = Build Array (concatenate)(w507, w506) -> (w505:i32[])
                    }
                  }
                }
              }
            }
          }
        }
        "Index" <- w400
        "Pulse No" <- w408
        n171 = Subtract(x=w414, y=3) -> (x-y=w422:i32)
        n172 = Array Subset(array=w421, index=w422) -> (→"subarray":bool[])  [unwired: 1 in]
        n173 = Subtract(x=w413, y=w414) -> (x-y=→"Last index":i32)
      }
      frame "Prepare Phase Lock Channels" {
        n174 = local read "Laser Status Index"() -> (w513:i32)
        n175 = local read "Laser Disp Index"() -> (w517:i32)
        n176 = Greater Or Equal To 0?(x=w517) -> (x >= 0?=w519:bool)
        n177 = case shown="False" w519 {
          tunnel: "Channel to Phase lock" -> [w533 w540]
          tunnel: w517 -> [_ w539]
          tunnel: [w533 w536] -> w514
          tunnel: w513 -> [_ w534]
          frame False {
          }
          frame True {
            n178 = Search 1D Array(1D array=w540, element=w539) -> (index of element=w542:i32)  [unwired: 1 in]
            n179 = Less Than 0?(x=w542) -> (x < 0?=w541:bool)
            n180 = case shown="True" w541 {
              tunnel: w540 -> [w548 w552]
              tunnel: w539 -> [_ w551]
              tunnel: [w548 w549] -> w535
              frame False {
              }
              frame True {
                n181 = Build Array (concatenate)(w552, w551) -> (w550:i32[])
                n182 = Sort 1D Array(array=w550) -> (sorted array=w549:i32[])
              }
            }
            n183 = Search 1D Array(1D array=w535, element=w534) -> (index of element=w537:i32)  [unwired: 1 in]
            n184 = Less Than 0?(x=w537) -> (x < 0?=w538:bool)
            n185 = case shown="True" w538 {
              tunnel: w535 -> [w543 w547]
              tunnel: w534 -> [_ w546]
              tunnel: [w543 w544] -> w536
              frame False {
              }
              frame True {
                n186 = Build Array (concatenate)(w547, w546) -> (w545:i32[])
                n187 = Sort 1D Array(array=w545) -> (sorted array=w544:i32[])
              }
            }
          }
        }
        n188 = for {
          tunnel: w514 -> [w562] mode=indexing
          tunnel: w532 -> [w561]
          shift-right: [w555] -> w511
          shift-left: dbl[][] [] -> [w556]
          shift-right: [w557] -> w526
          shift-left: i32[] [] -> [w558]
          i -> [w554]
          n189 = Index Array(array=w561, index=w562) -> (element=w560:T1)
          n190 = Unbundle By Name(w560) -> ("Eng Values"=w553:dbl[], "Inst Array"=w559:T3)
          n191 = case shown="\"Analogue\"" w559 {
            tunnel: w554 -> [_ w568 _]
            tunnel: w558 -> [w564 w567 w570]
            tunnel: [w564 w566 w570] -> w557
            tunnel: w556 -> [w563 w565 w572]
            tunnel: [w563 w565 w571] -> w555
            tunnel: w553 -> [_ _ w569]
            frame "PWA" {
            }
            frame "LDA" {
              n192 = Build Array (concatenate)(w567, w568) -> (w566:i32[])
            }
            frame "Analogue" {
              n193 = Build Array (concatenate)(w572, w569) -> (w571:dbl[][])
            }
          }
        }
        "LDA Chs" <- w526
        n194 = Search 1D Array(1D array=w514, element=w517) -> (index of element=→"Laser Phase lock index":i32)  [unwired: 1 in]
        n195 = Search 1D Array(1D array=w514, element=w513) -> (index of element=→"L Status Phase lock index":i32)  [unwired: 1 in]
        n196 = Array Size(array=w526) -> (size(s)=w527:i32)
        n197 = Greater Than 0?(x=w527) -> (x > 0?=w525:bool)
        n198 = Select(t="Produce Uniform LDA data", s=w525, f="WT trace Phase locked data") -> (s? t:f=w524:string)
      }
      frame "Produce Uniform LDA data" {
        n199 = Reciprocal(x=w591) -> (1/x=w592:dbl)
        n200 = Multiply(x=w592, y=1000.0) -> (x*y=w589:dbl)
        n201 = Array Size(array=w588) -> (size(s)=w587:i32[])
        n202 = Index Array(array=w587, index=1) -> (element=w585:i32)
        n203 = disable-structure shown="Enabled" {
          disable-tunnel: [w598 dbl[][] []] -> w582
          frame Disabled {
            n204 = global read "Plug_in_data_global.vi" "Vari Spaced"() -> (w598)
          }
          frame Enabled {
          }
        }
        n205 = for {
          N: w585 -> [_]
          tunnel: w589 -> [w609]
          tunnel: w576 -> [w608]
          tunnel: [w607] -> w584 mode=indexing
          i -> [w610]
          n206 = Multiply(x=w609, y=w610) -> (x*y=w606:dbl)
          n207 = Threshold 1D Array(2:w606, 3:w608) -> (0:w607:dbl)  [unwired: 1 out]
        }
        n208 = local read "LDA Chs"() -> (w583:i32[])
        n209 = for {
          tunnel: w583 -> [w613] mode=indexing
          tunnel: w582 -> [w612]
          tunnel: [w611] -> w581 mode=indexing
          n210 = Index Array(array=w612, index (row)=w613) -> (element=w611:dbl[])  [unwired: 1 in]
        }
        n211 = for {
          tunnel: [w602] -> w580 mode=indexing
          tunnel: w581 -> [w601] mode=indexing
          tunnel: w584 -> [w600]
          n212 = for {
            tunnel: [w605] -> w602 mode=indexing
            tunnel: w601 -> [w604]
            tunnel: w600 -> [w603] mode=indexing
            n213 = Interpolate 1D Array(1:w603, 2:w604) -> (0:w605:dbl)
          }
        }
        n214 = Build Array (concatenate)(w580, w579) -> (w577:dbl[][])
      }
      frame "WT trace Phase locked data" {
        n215 = local read "Index"() -> (w635:i32[])
        n216 = local read "WT trace index"() -> (w619:dbl[][])
        n217 = local read "Turbine to Phase Lock to"() -> (w618:u16)
        n218 = local read "Number of Revs"() -> (w636:i32)
        n219 = Array Subset(array=w635, index=1) -> (w641:i32[])  [unwired: 1 in]
        n220 = Index Array(array=w635, index=0) -> (element=w640:i32)
        n221 = Index Array(array=w619, index (row)=w618) -> (element=w617:dbl[])  [unwired: 1 in]
        n222 = Array Size(array=w641) -> (size(s)=w622:i32)
        "Last Block No of Revs" <- w622
        n223 = case shown="2, Default" w642 {
          tunnel: [w647 w652] -> w634
          tunnel: w622 -> [w648 w652]
          tunnel: w636 -> [w649 _]
          tunnel: [FALSE TRUE] -> w639
          tunnel: [w645 i32[] []] -> w625
          tunnel: w624 -> [w645 _]
          frame 2, Default {
            n224 = Add(x=w649, y=w648) -> (x+y=w647:i32)
          }
          frame 1 {
          }
        }
        "Number of Revs" <- w634
        n225 = Build Array (concatenate)(w617, w628) -> (w629:dbl[][])
        n226 = Increment(x=w627) -> (x+1=w626:dbl)
        n227 = for {
          shift-right: [w668] -> _
          shift-left: w640 -> [w661]
          tunnel: w641 -> [w668] mode=indexing
          tunnel: w639 -> [w665]
          shift-right: [w663] -> w637
          shift-left: w638 -> [w662]
          tunnel: w629 -> [w664]
          tunnel: w626 -> [w659]
          tunnel: w627 -> [w658]
          tunnel: [w655] -> w623 mode=indexing
          shift-right: [w653] -> w620
          shift-left: w621 -> [w654]
          i -> [w667]
          n228 = Subtract(x=w668, y=w661) -> (x-y=w655:i32)
          n229 = Equal To 0?(x=w667) -> (x = 0?=w666:bool)
          n230 = Divide(x=w655, y=w658) -> (x/y=w660:dbl)
          n231 = for {
            N: w659 -> [_]
            tunnel: w661 -> [w673]
            tunnel: w660 -> [w671]
            tunnel: [w669] -> w657 mode=indexing
            i -> [w672]
            n232 = Multiply(x=w671, y=w672) -> (x*y=w670:dbl)
            n233 = Add(x=w673, y=w670) -> (x+y=w669:dbl)
          }
          n234 = And(x=w665, y=w666) -> (x .and. y?=w656:bool)
          n235 = for {
            tunnel: w664 -> [w682] mode=indexing
            tunnel: w656 -> [w685]
            tunnel: [w684] -> w663 mode=indexing
            tunnel: w662 -> [w680]
            tunnel: w657 -> [w681]
            tunnel: w654 -> [w679]
            tunnel: [w676] -> w653 mode=indexing
            i -> [w678]
            # "u^2"
            # "U"
            n236 = for {
              tunnel: w682 -> [w688]
              tunnel: [w687] -> w677 mode=indexing
              tunnel: w681 -> [w686] mode=indexing
              n237 = Interpolate 1D Array(1:w686, 2:w688) -> (0:w687:dbl)
            }
            n238 = Index Array(array=w680, index (row)=w678) -> (element=w683:dbl[])  [unwired: 1 in]
            n239 = Index Array(array=w679, index (row)=w678) -> (element=w674:dbl[])  [unwired: 1 in]
            n240 = Multiply(x=w677, y=w677) -> (x*y=w675:dbl[])
            n241 = case shown="False" w685 {
              tunnel: [w694 w696] -> w684
              tunnel: w677 -> [w692 w696]
              tunnel: w683 -> [w693 _]
              tunnel: [w690 w695] -> w676
              tunnel: w675 -> [w691 w695]
              tunnel: w674 -> [w689 _]
              frame False {
                n242 = Add(x=w693, y=w692) -> (x+y=w694:dbl[])
                n243 = Add(x=w689, y=w691) -> (x+y=w690:dbl[])
              }
              frame True {
              }
            }
          }
        }
        n244 = Build Array (concatenate)(w625, w623) -> (w633:i32[])
      }
      frame "Output WT Statistics" {
        w713 = string[] []
        n245 = local read "All WTs"() -> (w715:dbl[][])
        n246 = for {
          tunnel: w715 -> [w727] mode=indexing
          shift-right: [w721] -> w714
          shift-left: w713 -> [w722]
          shift-right: [w717] -> w711
          shift-left: w713 -> [w719]
          tunnel: string[] ["WT_%d:Hub_RPM:Mean", "WT_%d:Hub_RPM:St_Dev", "WT_%d:Hub_RPM:Max-Min", "WT_%d:Number_of:Revs"] ("Plug in titles") -> [w720]
          i -> [w716]
          n247 = Index Array(array=w727, index=0) -> (element=w726:dbl)
          n248 = Index Array(array=w727, index=1) -> (element=w725:dbl)
          n249 = Index Array(array=w727, index=2) -> (element=w724:dbl)
          n250 = Index Array(array=w727, index=3) -> (element=w723:dbl)
          n251 = for {
            tunnel: w720 -> [w739] mode=indexing
            tunnel: [w737] -> w718 mode=indexing
            tunnel: w716 -> [w736]
            n252 = Increment(x=w736) -> (x+1=w738:i32)
            n253 = Format Into String(format string=w739, w738) -> (resulting string=w737:string)  [unwired: 2 in, 1 out]
          }
          n254 = call "Number_2_string.vi"("number"=w726) -> ("String"=w734:string)  [unwired: 1 in]
          n255 = call "Number_2_string.vi"("number"=w725) -> ("String"=w735:string)  [unwired: 1 in]
          n256 = call "Number_2_string.vi"("number"=w724) -> ("String"=w733:string)  [unwired: 1 in]
          n257 = Number To Decimal String(number=w723) -> (decimal integer string=w732:string)  [unwired: 1 out]
          n258 = Build Array (concatenate)(w722, w734, w735, w733, w732) -> (w721:string[])
          n259 = Build Array (concatenate)(w719, w718) -> (w717:string[])
        }
        "Plug in titles" <- w711
        "Plug in values" <- w714
        n260 = local read "Laser Disp Index"() -> (w709:i32)
        n261 = Greater Or Equal To 0?(x=w709) -> (x >= 0?=w708:bool)
        n262 = Select(t="Laser Displacement Analysis", s=w708, f="Get Last Block info") -> (s? t:f=w707:string)
      }
      frame "Laser Displacement Analysis" {
        # "D^2"
        # "D"
        n263 = stacked-sequence {
          seq-local: [_ w770 _ _ _] -> [_ _ w784 _ _]
          seq-local: [_ _ w785 _ _] -> [_ _ _ w825 _]
          seq-local: [w760 _ _ _ _] -> [_ _ _ w821 _]
          seq-local: [w757 _ _ _ _] -> [_ _ _ w820 _]
          tunnel: w753 -> [_ _ _ _ _]
          tunnel: w752 -> [_ _ _ _ _]
          tunnel: w749 -> [w767 w775 _ _ _]
          tunnel: w748 -> [_ _ _ _ _]
          tunnel: w747 -> [_ _ _ w819 _]
          tunnel: w746 -> [w768 _ _ _ _]
          tunnel: w745 -> [_ _ _ _ w888]
          tunnel: [_ _ _ _ TRUE] -> w744
          tunnel: [_ _ _ _ "Get Last Block info"] -> w743
          frame #0 {
            n264 = local read "Laser Phase lock index"() -> (w759:i32)
            n265 = local read "Number of Revs"() -> (w763:i32)
            n266 = Increment(x=w759) -> (x+1=w756:i32)
            n267 = Index Array(array=w768, index (row)=w756) -> (element=w765:dbl[])  [unwired: 1 in]
            n268 = Index Array(array=w767, index (row)=w756) -> (element=w764:dbl[])  [unwired: 1 in]
            n269 = Divide(x=w765, y=w763) -> (x/y=w754:dbl[])
            n270 = Divide(x=w764, y=w763) -> (x/y=w755:dbl[])
            "Waveform Graph 3" <- w755
            n271 = Build Array (concatenate)(w755, w755, 0.0) -> (w757:dbl[])
            n272 = Square(x=w755) -> (x^2=w766:dbl[])
            n273 = Subtract(x=w754, y=w766) -> (x-y=w762:dbl[])
            n274 = Build Array (concatenate)(w762, w762, 0.0) -> (w760:dbl[])
          }
          frame #1 {
            n275 = local read "L Status Phase lock index"() -> (w776:i32)
            n276 = local read "Number of Revs"() -> (w778:i32)
            n277 = Increment(x=w776) -> (x+1=w777:i32)
            n278 = Index Array(array=w775, index (row)=w777) -> (element=w779:dbl[])  [unwired: 1 in]
            n279 = Divide(x=w779, y=w778) -> (x/y=w773:dbl[])
            n280 = Build Array (concatenate)(w773, w773, 0.0) -> (w772:dbl[])
            n281 = Greater?(x=w772, y=0.4) -> (0:w770:bool[])
            n282 = Array Size(array=w770) -> (size(s)=w769:i32)
            n283 = Divide(x=w769, y=2) -> (x/y=w782:dbl)
            n284 = Boolean To (0,1)(Boolean=w770) -> (0, 1=w783:i16[])
            n285 = Array Subset(array=w783, length=w782) -> (→"Waveform Graph 2":i16[])  [unwired: 1 in]
          }
          frame #2 {
            n286 = Index Array(array=w784, index=0) -> (element=w787:bool)
            n287 = for {
              tunnel: w784 -> [w794] mode=indexing
              shift-right: [w794] -> _
              shift-left: w787 -> [w789]
              shift-right: [w791] -> w785
              shift-left: i32[] [] -> [w792]
              i -> [w793]
              n288 = Not Equal?(x=w794, y=w789) -> (x != y?=w790:bool)
              n289 = case shown="True" w790 {
                tunnel: w793 -> [_ w801]
                tunnel: w792 -> [w795 w799]
                tunnel: [w795 w800] -> w791
                tunnel: w789 -> [_ w796]
                frame False {
                }
                frame True {
                  n290 = Array Size(array=w799) -> (size(s)=w798:i32)
                  n291 = Equal To 0?(x=w798) -> (x = 0?=w797:bool)
                  n292 = case shown="False" w797 {
                    tunnel: w801 -> [w802 w808]
                    tunnel: w799 -> [w804 w807]
                    tunnel: [w803 w806] -> w800
                    tunnel: w796 -> [_ w805]
                    frame False {
                      n293 = Build Array (concatenate)(w804, w802) -> (w803:i32[])
                    }
                    frame True {
                      n294 = case shown="False" w805 {
                        tunnel: w808 -> [_ w812]
                        tunnel: w807 -> [w809 w811]
                        tunnel: [w809 w810] -> w806
                        frame False {
                        }
                        frame True {
                          n295 = Build Array (concatenate)(w811, w812) -> (w810:i32[])
                        }
                      }
                    }
                  }
                }
              }
            }
            "Array" <- w785
          }
          frame #3 {
            w814 = 360.0 ("y")
            n296 = Divide(x="Start Cut Deg", y=w819) -> (x/y=w827:dbl)
            n297 = Divide(x="End Cut Deg", y=w819) -> (x/y=w828:dbl)
            n298 = To Long Integer(number=w827) -> (32bit integer=w823:i32)
            n299 = To Long Integer(number=w828) -> (32bit integer=w826:i32)
            n300 = Add(x=w823, y=w826) -> (x+y=w822:i32)
            n301 = global read "Wind_Turbine_Global.vi" "Radius (mm)"() -> (w813:dbl)
            n302 = Divide(x=w819, y=w814) -> (x/y=w818:dbl)
            n303 = Multiply(x=w818, y=6.283185307179586) -> (x*y=w817:dbl)
            n304 = Multiply(x=w817, y=w813) -> (x*y=w815:dbl)
            n305 = for {
              N: 3 -> [_]
              tunnel: w820 -> [w861]
              tunnel: w825 -> [w858]
              tunnel: w823 -> [w854]
              tunnel: w822 -> [w853]
              tunnel: w815 -> [w852]
              tunnel: w821 -> [w843]
              tunnel: w814 -> [w836]
              i -> [w851]
              n306 = Multiply(x=w851, y=2) -> (x*y=w856:i32)
              n307 = Increment(x=w856) -> (x+1=w855:i32)
              n308 = Index Array(array=w858, index=w856) -> (element=w863:i32)
              n309 = Index Array(array=w858, index=w855) -> (element=w864:i32)
              n310 = Subtract(x=w864, y=w863) -> (x-y=w862:i32)
              n311 = Add(x=w863, y=w854) -> (x+y=w846:i32)
              n312 = Subtract(x=w862, y=w853) -> (x-y=w848:i32)
              n313 = Array Subset(array=w843, index=w846, length=w848) -> (w834:dbl[])
              n314 = call <vilib>:"Mean.vi"("X"=w834) -> ("mean"=w833:dbl)  [unwired: 1 out]
              n315 = Multiply(x=2.0, y=w833) -> (x*y=w831:dbl)
              n316 = call "Top_and_Tail_ph.vi"("Array in"=w834, "Threshold"=w831) -> ("Length"=w841:i32, "Start Index"=w845:i32)
              n317 = Add(x=w846, y=w845) -> (x+y=w842:i32)
              n318 = Array Subset(array=w843, index=w842, length=w841) -> (w844:dbl[])
              n319 = call <vilib>:"Mean.vi"("X"=w844) -> ("mean"=w847:dbl)  [unwired: 1 out]
              n320 = Array Subset(array=w861, index=w842, length=w841) -> (w850:dbl[])
              n321 = Array Size(array=w850) -> (size(s)=w860:i32)
              n322 = for {
                N: w860 -> [_]
                tunnel: w852 -> [w885]
                tunnel: [w883] -> w859 mode=indexing
                i -> [w884]
                n323 = Multiply(x=w884, y=w885) -> (x*y=w883:dbl)
              }
              n324 = call <vilib>:"Linear Fit.vi"("Y"=w850, "X"=w859) -> ("slope"=w840:dbl)  [unwired: 9 in, 4 out]
              n325 = call <vilib>:"Mean.vi"("X"=w850) -> ("mean"=w849:dbl)  [unwired: 1 out]
              n326 = Inverse Tangent(1:w840) -> (0:w839:dbl)
              n327 = Divide(x=w839, y=6.283185307179586) -> (x/y=w837:dbl)
              n328 = Multiply(x=w837, y=w836) -> (x*y=w835:dbl)
              n329 = case shown="2" w851 {
                tunnel: w850 -> [w870 w873 w879]
                tunnel: w840 -> [w869 w875 w881]
                tunnel: w849 -> [w868 w876 w882]
                tunnel: w844 -> [w867 w874 w880]
                tunnel: w847 -> [w866 w872 w878]
                tunnel: w835 -> [w865 w871 w877]
                frame 0, Default {
                  "slope 1" <- w869
                  "Mean Blade 1" <- w870
                  "Av Disp 1" <- w868
                  "Variance Blade 1" <- w867
                  "Av Variance 1" <- w866
                  "Angle 1" <- w865
                }
                frame 1 {
                  "Av Disp 2" <- w876
                  "Mean Blade 2" <- w873
                  "Variance Blade 2" <- w874
                  "slope 2" <- w875
                  "Av Variance 2" <- w872
                  "Angle 2" <- w871
                }
                frame 2 {
                  "Av Disp 3" <- w882
                  "Mean Blade 3" <- w879
                  "Variance Blade 3" <- w880
                  "slope 3" <- w881
                  "Av Variance 3" <- w878
                  "Angle 3" <- w877
                }
              }
            }
          }
          frame #4 {
            n330 = case shown="True" w888 {
              frame False {
              }
              frame True {
                n331 = for {
                  N: 3 -> [_]
                  tunnel: [w919] -> w910 mode=indexing
                  tunnel: [w918] -> w909 mode=indexing
                  tunnel: [w917] -> w908 mode=indexing
                  tunnel: [w916] -> w892 mode=indexing
                  i -> [w925]
                  n332 = Increment(x=w925) -> (x+1=w924:i32)
                  n333 = Format Into String(format string="Blade %d:", w924) -> (resulting string=w915:string)  [unwired: 2 in, 1 out]
                  n334 = Concatenate Strings(w915, "Angle:") -> (w916:string)
                  n335 = Concatenate Strings(w915, "Slope:") -> (w919:string)
                  n336 = Concatenate Strings(w915, "Average:X") -> (w918:string)
                  n337 = Concatenate Strings(w915, "Variance of:X") -> (w917:string)
                }
                n338 = local read "Av Variance 1"() -> (w899:dbl)
                n339 = local read "Av Variance 2"() -> (w898:dbl)
                n340 = local read "Av Variance 3"() -> (w897:dbl)
                n341 = local read "Av Disp 1"() -> (w902:dbl)
                n342 = local read "Av Disp 2"() -> (w901:dbl)
                n343 = local read "Av Disp 3"() -> (w900:dbl)
                n344 = local read "slope 1"() -> (w905:dbl)
                n345 = local read "slope 2"() -> (w904:dbl)
                n346 = local read "slope 3"() -> (w903:dbl)
                n347 = local read "Angle 3"() -> (w891:dbl)
                n348 = local read "Angle 1"() -> (w890:dbl)
                n349 = local read "Angle 2"() -> (w889:dbl)
                n350 = Build Array(w890, w889, w891, w905, w904, w903, w902, w901, w900, w899, w898, w897) -> (w896:dbl[])
                n351 = local read "Plug in values"() -> (w895:string[])
                n352 = local read "Plug in titles"() -> (w907:string[])
                n353 = for {
                  tunnel: w896 -> [w913] mode=indexing
                  tunnel: [w912] -> w894 mode=indexing
                  n354 = call "Number_2_string.vi"("number"=w913) -> ("String"=w912:string)  [unwired: 1 in]
                }
                n355 = Build Array (concatenate)(w907, w892, w910, w909, w908) -> (w906:string[])
                n356 = Build Array (concatenate)(w895, w894) -> (w893:string[])
                n357 = local write "Plug in titles"(w906) -> ()
                n358 = local write "Plug in values"(w893) -> ()
              }
            }
          }
        }
      }
      frame "Get Last Block info" {
        n359 = case shown="\"Take New Data\"" w937 {
          tunnel: w939 -> [_ _]
          tunnel: w938 -> [_ _]
          tunnel: [w940 "Post Process"] -> w936
          tunnel: [w944 TRUE ("Processing last block?")] -> w930
          tunnel: w929 -> [w944 _]
          frame "Take New Data" {
            n360 = Select(t="Change Dem Volts", s="Change Dem Voltages?", f="Post Process") -> (s? t:f=w940:string)
          }
          frame "Post Process Raw Data File" {
          }
        }
      }
      frame "Change Dem Volts" {
        n361 = local read "All WTs"() -> (w971:dbl[][])
        n362 = for {
          tunnel: w975 -> [w1003]
          tunnel: [w1002] -> w974 mode=indexing
          tunnel: [w1001] -> w957 mode=indexing
          tunnel: w971 -> [w999] mode=indexing
          tunnel: [w998] -> w969 mode=indexing
          tunnel: [w997] -> w951
          tunnel: w950 -> [w996]
          i -> [w1004]
          n363 = Increment(x=w1004) -> (x+1=w997:i32)
          n364 = Format Into String(format string=w1003, w997) -> (resulting string=w1001:string)  [unwired: 2 in, 1 out]
          n365 = Format Into String(format string=w996, w997) -> (resulting string=w1002:string)  [unwired: 2 in, 1 out]
          n366 = Index Array(array=w999, index=0) -> (element=w998:dbl)
        }
        n367 = Build Array (concatenate)(w974, w957) -> (w973:string[])
        n368 = call "Get_Current_Scan_client.vi"("ADAM Ch Names"=w973) -> ("Numerical Values"=w972:dbl[])  [unwired: 3 out]
        n369 = Split 1D Array(array=w972, index=w951) -> (first subarray=w970:dbl[], second subarray=w968:dbl[])
        n370 = Divide(x=w970, y=w969) -> (x/y=w960:dbl[])
        n371 = In Range and Coerce(upper limit=1.05, x=w960, lower limit=0.95) -> (coerced(x)=w959:dbl[], In Range?=w958:bool[])
        n372 = Multiply(x=w959, y=w968) -> (x*y=w963:dbl[])
        n373 = In Range and Coerce(upper limit=9.9, x=w963, lower limit=0.0) -> (coerced(x)=w956:dbl[])  [unwired: 1 out]
        n374 = for {
          shift-right: [w985] -> w954
          shift-left: string[] [] -> [w986]
          shift-right: [w983] -> w955
          shift-left: dbl[] [] -> [w984]
          tunnel: w958 -> [w987] mode=indexing
          tunnel: w957 -> [w982] mode=indexing
          tunnel: w956 -> [w981] mode=indexing
          n375 = case shown="False" w987 {
            tunnel: w986 -> [w989 w995]
            tunnel: [w989 w994] -> w985
            tunnel: w984 -> [w988 w993]
            tunnel: [w988 w992] -> w983
            tunnel: w982 -> [_ w991]
            tunnel: w981 -> [_ w990]
            frame False {
            }
            frame True {
              n376 = Build Array (concatenate)(w995, w991) -> (w994:string[])
              n377 = Build Array (concatenate)(w993, w990) -> (w992:dbl[])
            }
          }
        }
        n378 = call "ASYNC_Adam_client.vi"("Values"=w955, "Channel Names"=w954) -> ()  [unwired: 2 out]
      }
      frame "Post Process" {
        n379 = Compound Arithmetic op=AND("Add Phase data to results file", w1012) -> (w1011:bool)
        n380 = case shown="True" w1011 {
          tunnel: w1010 -> [_ w1022]
          tunnel: w1009 -> [_ w1021]
          tunnel: w1008 -> [_ w1020]
          frame False {
          }
          frame True {
            n381 = stacked-sequence {
              tunnel: w1022 -> [w1024 _]
              tunnel: w1021 -> [_ w1051]
              tunnel: w1020 -> [_ w1055]
              frame #0 {
                n382 = local read "Channel to Phase lock"() -> (w1031:i32[])
                n383 = property on="Channel to Phase lock" class="LstBox (strict)"() -> ("Item Names"=w1030:string[])  [unwired: 2 in, 2 out]
                n384 = local read "Plug in titles"() -> (w1025:string[])
                n385 = Divide(x=360, y=w1024) -> (x/y=w1027:dbl)
                n386 = Increment(x=w1024) -> (x+1=w1023:dbl)
                n387 = for {
                  tunnel: w1030 -> [w1049]
                  tunnel: w1031 -> [w1048] mode=indexing
                  tunnel: [w1047] -> w1029 mode=indexing
                  n388 = Index Array(array=w1049, index=w1048) -> (element=w1047:string)
                }
                n389 = for {
                  tunnel: w1029 -> [w1038] mode=indexing
                  tunnel: w1027 -> [w1037]
                  shift-right: [w1034] -> w1026
                  shift-left: w1025 -> [w1036]
                  tunnel: w1023 -> [w1032]
                  n390 = for {
                    N: w1032 -> [_]
                    tunnel: w1038 -> [w1041]
                    tunnel: w1037 -> [w1045]
                    tunnel: [w1043] -> w1035 mode=indexing
                    tunnel: [w1040] -> w1033 mode=indexing
                    i -> [w1046]
                    n391 = Multiply(x=w1045, y=w1046) -> (x*y=w1039:dbl)
                    n392 = Format Into String(format string="%s:Mean:%.1f Deg:%.1f", w1041, w1039, w1039) -> (resulting string=w1043:string)  [unwired: 2 in, 1 out]
                    n393 = Format Into String(format string="%s:Variance:%.1f Deg:%.1f", w1041, w1039, w1039) -> (resulting string=w1040:string)  [unwired: 2 in, 1 out]
                  }
                  n394 = Build Array (concatenate)(w1036, w1035, w1033) -> (w1034:string[])
                }
                n395 = local write "Plug in titles"(w1026) -> ()
              }
              frame #1 {
                n396 = local read "Number of Revs"() -> (w1058:i32)
                n397 = Array Subset(array=w1055, index (row)=1 ("index")) -> (w1053:dbl[][])  [unwired: 3 in]
                n398 = Array Subset(array=w1051, index (row)=1 ("index")) -> (w1050:dbl[][])  [unwired: 3 in]
                n399 = local read "Plug in values"() -> (w1060:string[])
                n400 = Divide(x=w1050, y=w1058) -> (x/y=w1059:dbl[][])
                n401 = Divide(x=w1053, y=w1058) -> (x/y=w1056:dbl[][])
                n402 = for {
                  tunnel: w1059 -> [w1066] mode=indexing
                  shift-right: [w1064] -> w1057
                  shift-left: w1060 -> [w1065]
                  tunnel: w1056 -> [w1062] mode=indexing
                  n403 = for {
                    tunnel: w1066 -> [w1071] mode=indexing
                    tunnel: [w1072] -> w1063 mode=indexing
                    tunnel: w1062 -> [w1070] mode=indexing
                    tunnel: [w1067] -> w1061 mode=indexing
                    n404 = Multiply(x=w1071, y=w1071) -> (x*y=w1069:dbl)
                    n405 = Subtract(x=w1070, y=w1069) -> (x-y=w1068:dbl)
                    n406 = call "Number_2_string.vi"("number"=w1071) -> ("String"=w1072:string)  [unwired: 1 in]
                    n407 = call "Number_2_string.vi"("number"=w1068) -> ("String"=w1067:string)  [unwired: 1 in]
                  }
                  n408 = Build Array (concatenate)(w1065, w1063, w1061) -> (w1064:string[])
                }
                n409 = local write "Plug in values"(w1057) -> ()
              }
            }
          }
        }
        n410 = Compound Arithmetic op=AND("Save Phase averaged Profiles", w1012) -> (w1014:bool)
      }
      frame "Check Folder Name" {
        n411 = File/Directory Info(path="Output Directory") -> (error out=w1081:errorcluster)  [unwired: 1 in, 6 out]
        n412 = Empty String/Path?(string/path="Output Directory") -> (empty?=w1083:bool)
        n413 = Unbundle By Name(w1081) -> ("status"=w1082:bool)
        n414 = Or(x=w1083, y=w1082) -> (x .or. y?=w1084:bool)
        n415 = case shown="True" w1084 {
          tunnel: [w1091 w1097] -> w1077
          tunnel: "Output Directory" -> [w1091 w1095]
          tunnel: [FALSE ("cancelled") w1092] -> w1079
          frame False {
          }
          frame True {
            n416 = Strip Path(path=w1095) -> (stripped path=w1094:path, name=w1093:string)
            n417 = File Dialog(7:"Please Select a new or existing Results folder" ("prompt"), 9:w1093, 11:w1094) -> (1:w1092:bool, 3:w1097:path)  [unwired: 1 in, 5 out]
          }
        }
        n418 = local write "Output Directory"(w1077) -> ()
        n419 = Not(x=w1079) -> (.not. x?=w1078:bool)
      }
      frame "Save Phase locked data" {
        n420 = global read "Meas_global.vi" "Raw data file"() -> (w1105:path)
        n421 = stacked-sequence {
          seq-local: [_ w1148 _ _] -> [_ _ _ w1205]
          seq-local: [w1122 _ _ _] -> [_ _ _ w1206]
          seq-local: [_ _ w1164 _] -> [_ _ _ w1204]
          seq-local: [w1111 _ _ _] -> [_ _ w1162 _]
          tunnel: w1107 -> [_ _ _ _]
          tunnel: w1105 -> [w1121 _ _ w1210]
          tunnel: w1103 -> [w1118 _ _ _]
          tunnel: w1102 -> [w1117 _ _ _]
          tunnel: w1101 -> [_ _ w1161 _]
          frame #0 {
            w1123 = "\r\n"
            n422 = local read "Number of Revs"() -> (w1116:i32)
            n423 = Array Subset(array=w1117, index (row)=1 ("index")) -> (w1114:dbl[][])  [unwired: 3 in]
            n424 = Array Subset(array=w1118, index (row)=1 ("index")) -> (w1115:dbl[][])  [unwired: 3 in]
            n425 = for {
              tunnel: w1116 -> [w1131]
              tunnel: w1115 -> [w1130] mode=indexing
              tunnel: w1114 -> [w1129] mode=indexing
              tunnel: [w1127] -> w1113 mode=indexing
              tunnel: [w1126] -> w1112 mode=indexing
              n426 = Divide(x=w1130, y=w1131) -> (x/y=w1127:dbl[])
              n427 = Divide(x=w1129, y=w1131) -> (x/y=w1128:dbl[])
              n428 = Multiply(x=w1127, y=w1127) -> (x*y=w1132:dbl[])
              n429 = Subtract(x=w1128, y=w1132) -> (x-y=w1126:dbl[])
            }
            n430 = call "Read_RD_Ch_header.vi"("Raw data file"=w1121) -> ("Ch string"=w1125:string)  [unwired: 3 out]
            n431 = Build Array (concatenate)(w1113, w1112) -> (w1111:dbl[][])
            n432 = Concatenate Strings(w1123, "*****This is a many rows per single point file*****", w1123, w1125) -> (w1122:string)
          }
          frame #1 {
            w1134 = "\r\n"
            n433 = local read "Channel to Phase lock"() -> (w1150:i32[])
            n434 = property on="Channel to Phase lock" class="LstBox (strict)"() -> ("Item Names"=w1149:string[])  [unwired: 2 in, 2 out]
            n435 = Initialize Array("", 10) -> (w1151:string[])
            n436 = call "Asterisk_header.vi"("Channel names"=w1151) -> ("Header string"=w1133:string)
            n437 = for {
              tunnel: w1150 -> [w1159] mode=indexing
              tunnel: w1149 -> [w1158]
              tunnel: [w1157] -> w1146 mode=indexing
              tunnel: ["Mean" ("format string")] -> w1144 mode=indexing
              tunnel: ["Variance" ("format string")] -> w1143 mode=indexing
              tunnel: [""] -> w1141 mode=indexing
              n438 = Index Array(array=w1158, index=w1159) -> (element=w1157:string)
            }
            n439 = Build Array (concatenate)("Rotor", w1146, w1146) -> (w1140:string[])
            n440 = Build Array (concatenate)("Angle", w1144, w1143) -> (w1139:string[])
            n441 = Build Array (concatenate)("(deg)", w1141, w1141) -> (w1138:string[])
            n442 = Build Array(w1140, w1139, w1138) -> (w1137:string[][])
            n443 = Array To Spreadsheet String(array=w1137, 3:"%s" ("format string")) -> (spreadsheet string=w1135:string)  [unwired: 1 out]
            n444 = Concatenate Strings(w1134, w1133, w1135, w1134) -> (w1148:string)
          }
          frame #2 {
            n445 = Array Size(array=w1162) -> (size(s)=w1165:i32[])
            n446 = Index Array(array=w1165, index=0) -> (element=w1171:i32)
            n447 = Divide(x=360, y=w1161) -> (x/y=w1160:dbl)
            n448 = Index Array(array=w1165, index=1) -> (element=w1166:i32)
            n449 = Decrement(x=w1171) -> (x-1=w1172:i32)
            n450 = for {
              N: w1166 -> [_]
              shift-right: [w1185] -> w1164
              shift-left: "" -> [w1180]
              tunnel: "Separation Character" -> [w1176]
              tunnel: w1162 -> [w1183]
              tunnel: w1172 -> [w1179]
              tunnel: w1160 -> [w1178]
              i -> [w1175]
              n451 = Index Array(array=w1183, index (col)=w1175) -> (element=w1182:dbl[])  [unwired: 1 in]
              n452 = Multiply(x=w1175, y=w1178) -> (x*y=w1174:dbl)
              n453 = call "Number_2_string.vi"("number"=w1174) -> ("String"=w1173:string)  [unwired: 1 in]
              n454 = Concatenate Strings(w1173, w1176) -> (w1177:string)
              n455 = for {
                shift-right: [w1193] -> w1181
                shift-left: w1177 -> [w1194]
                tunnel: w1176 -> [w1192]
                tunnel: w1182 -> [w1188] mode=indexing
                tunnel: w1179 -> [w1190]
                i -> [w1191]
                n456 = Equal?(x=w1191, y=w1190) -> (x = y?=w1189:bool)
                n457 = call "Number_2_string.vi"("precision"="precision", "number"=w1188) -> ("String"=w1187:string)
                n458 = case shown="False" w1189 {
                  tunnel: w1194 -> [w1198 w1201]
                  tunnel: w1187 -> [w1197 w1200]
                  tunnel: [w1196 w1199] -> w1193
                  tunnel: w1192 -> [w1195 _]
                  frame False {
                    n459 = Concatenate Strings(w1198, w1197, w1195) -> (w1196:string)
                  }
                  frame True {
                    n460 = Concatenate Strings(w1201, w1200) -> (w1199:string)
                  }
                }
              }
              n461 = Concatenate Strings(w1180, w1181, "\r\n") -> (w1185:string)
            }
          }
          frame #3 {
            w1202 = FALSE  # append to file? (new file:F)
            n462 = Strip Path(path=w1210) -> (name=w1208:string)  [unwired: 1 out]
            n463 = local read "Output Directory"() -> (w1209:path)
            n464 = Build Path(base path=w1209, name or relative path=w1208) -> (appended path=w1207:path)
            n465 = Concatenate Strings(w1206, w1205, w1204) -> (w1203:string)
            n466 = call "Write_File_Simple.vi"("append to file? (new file:F)"=w1202, "character string"=w1203, "file path"=w1207) -> ()  [unwired: 2 out]
          }
        }
      }
      frame "Save Phase locked data 1" {
        n467 = global read "Meas_global.vi" "Raw data file"() -> (w1218:path)
        n468 = stacked-sequence {
          seq-local: [_ w1251 _ _] -> [_ _ _ w1309]
          seq-local: [w1229 _ _ _] -> [_ _ _ w1310]
          seq-local: [_ _ w1265 _] -> [_ _ _ w1308]
          seq-local: [w1224 _ _ _] -> [_ _ w1264 _]
          tunnel: w1220 -> [_ _ _ _]
          tunnel: w1218 -> [w1228 _ _ w1314]
          tunnel: w1212 -> [w1227 _ _ _]
          tunnel: w1211 -> [_ _ w1263 _]
          frame #0 {
            w1230 = "\r\n"
            n469 = for {
              tunnel: w1227 -> [w1235] mode=indexing
              tunnel: [w1234] -> w1226 mode=indexing
              tunnel: [w1233] -> w1225 mode=indexing
              n470 = Unbundle(w1235) -> (w1234:dbl[], w1233:dbl[])
            }
            n471 = call "Read_RD_Ch_header.vi"("Raw data file"=w1228) -> ("Ch string"=w1232:string)  [unwired: 3 out]
            n472 = Concatenate Strings(w1230, "*****This is a many rows per single point file*****", w1230, w1232) -> (w1229:string)
            n473 = Build Array (concatenate)(w1226, w1225) -> (w1224:dbl[][])
          }
          frame #1 {
            w1237 = "\r\n"
            n474 = local read "Channel to Phase lock"() -> (w1253:i32[])
            n475 = property on="Channel to Phase lock" class="LstBox (strict)"() -> ("Item Names"=w1252:string[])  [unwired: 2 in, 2 out]
            n476 = Initialize Array("", 10) -> (w1254:string[])
            n477 = call "Asterisk_header.vi"("Channel names"=w1254) -> ("Header string"=w1236:string)
            n478 = for {
              tunnel: w1253 -> [w1262] mode=indexing
              tunnel: w1252 -> [w1261]
              tunnel: [w1260] -> w1249 mode=indexing
              tunnel: ["Mean" ("format string")] -> w1247 mode=indexing
              tunnel: ["Variance" ("format string")] -> w1246 mode=indexing
              tunnel: [""] -> w1244 mode=indexing
              n479 = Index Array(array=w1261, index=w1262) -> (element=w1260:string)
            }
            n480 = Build Array (concatenate)("Rotor", w1249, w1249) -> (w1243:string[])
            n481 = Build Array (concatenate)("Angle", w1247, w1246) -> (w1242:string[])
            n482 = Build Array (concatenate)("(deg)", w1244, w1244) -> (w1241:string[])
            n483 = Build Array(w1243, w1242, w1241) -> (w1240:string[][])
            n484 = Array To Spreadsheet String(array=w1240, 3:"%s" ("format string")) -> (spreadsheet string=w1238:string)  [unwired: 1 out]
            n485 = Concatenate Strings(w1237, w1236, w1238, w1237) -> (w1251:string)
          }
          frame #2 {
            n486 = Array Size(array=w1264) -> (size(s)=w1266:i32[])
            n487 = Index Array(array=w1266, index=0) -> (element=w1272:i32)
            n488 = Index Array(array=w1266, index=1) -> (element=w1267:i32)
            n489 = Decrement(x=w1272) -> (x-1=w1273:i32)
            n490 = for {
              N: w1267 -> [_]
              shift-right: [w1289] -> w1265
              shift-left: "" -> [w1284]
              tunnel: "Separation Character 2" -> [w1281]
              tunnel: w1264 -> [w1287]
              tunnel: w1273 -> [w1283]
              tunnel: w1263 -> [w1278]
              i -> [w1280]
              n491 = Index Array(array=w1287, index (col)=w1280) -> (element=w1286:dbl[])  [unwired: 1 in]
              n492 = Multiply(x=w1280, y=w1278) -> (x*y=w1275:dbl)
              n493 = Divide(x=w1278, y=2.0) -> (x/y=w1276:dbl)
              n494 = Add(x=w1275, y=w1276) -> (x+y=w1274:dbl)
              n495 = call "Number_2_string.vi"("number"=w1274) -> ("String"=w1279:string)  [unwired: 1 in]
              n496 = Concatenate Strings(w1279, w1281) -> (w1282:string)
              n497 = for {
                shift-right: [w1297] -> w1285
                shift-left: w1282 -> [w1298]
                tunnel: w1281 -> [w1296]
                tunnel: w1286 -> [w1292] mode=indexing
                tunnel: w1283 -> [w1294]
                i -> [w1295]
                n498 = Equal?(x=w1295, y=w1294) -> (x = y?=w1293:bool)
                n499 = call "Number_2_string.vi"("precision"="precision 2", "number"=w1292) -> ("String"=w1291:string)
                n500 = case shown="False" w1293 {
                  tunnel: w1298 -> [w1302 w1305]
                  tunnel: w1291 -> [w1301 w1304]
                  tunnel: [w1300 w1303] -> w1297
                  tunnel: w1296 -> [w1299 _]
                  frame False {
                    n501 = Concatenate Strings(w1302, w1301, w1299) -> (w1300:string)
                  }
                  frame True {
                    n502 = Concatenate Strings(w1305, w1304) -> (w1303:string)
                  }
                }
              }
              n503 = Concatenate Strings(w1284, w1285, "\r\n") -> (w1289:string)
            }
          }
          frame #3 {
            w1306 = FALSE  # append to file? (new file:F)
            n504 = Strip Path(path=w1314) -> (name=w1312:string)  [unwired: 1 out]
            n505 = local read "Output Directory"() -> (w1313:path)
            n506 = Build Path(base path=w1313, name or relative path=w1312) -> (appended path=w1311:path)
            n507 = Concatenate Strings(w1310, w1309, w1308) -> (w1307:string)
            n508 = call "Write_File_Simple.vi"("append to file? (new file:F)"=w1306, "character string"=w1307, "file path"=w1311) -> ()  [unwired: 2 out]
          }
        }
      }
    }
  }
